vi "Defect Buddy 2014-09-20.vi"() -> ()   [LabVIEW 2010]
uses:
  <vilib>/addons/database/Connection.llb/Conn ObjectReference.ctl
  <vilib>/addons/database/_DB Variant To Data/Database Variant To Data.xnode
  <vilib>/addons/database/Connection.llb/DB Tools Open Connec (Path).vi
  <vilib>/addons/database/Connection.llb/Conn Execute.vi
  <vilib>/addons/database/Recordset.llb/Rec Fetch Recordset Data (R).vi
  <vilib>/addons/database/Recordset.llb/Rec Destroy - Connection.vi
  <vilib>/Utility/file.llb/Write To Spreadsheet File (string).vi
  <vilib>/addons/database/NI_Database_API.lvlib
  <vilib>/picture/3D Picture Control/NI_3D Picture Control.lvlib
panel:
  in  "Volumes":dbl[](array[numeric])=[5230.5515143, 4360.60278, 2309.371815, 7792.576126]
  in  "Markov-Payne Correction":bool
  out "Loaded Structure":T1={"Structure Name"="Batch6_3+111 Quasi-Bulk", "Lattice vector a"=[9.1641, 0.0, 0.0], "Lattice vector b"=[0.0, 7.93635, 0.0], "Lattice vector c"=[0.0, 0.0, 53.7091], "Atoms Array"=[{"Atom Name"="", "Positions (Direct)"=[[0.036896, 0.129554, 0.035254], [0.536896, 0.129554, 0.035254], [0.286896, 0.629554, 0.035254], [0.786896, 0.629554, 0.035254], [0.285415, 0.295133, 0.107673], [0.785415, 0.295133, 0.107673], [0.035415, 0.795133, 0.107673], [0.535415, 0.795133, 0.107673], [0.033615, 0.463308, 0.180101], [0.533615, 0.463308, 0.180101], [0.283615, 0.963308, 0.180101], [0.783615, 0.963308, 0.180101], [0.030844, 0.131453, 0.252535], [0.530844, 0.131453, 0.252535], [0.280844, 0.631453, 0.252535], [0.780844, 0.631453, 0.252535], [0.278379, 0.302058, 0.324923], [0.778379, 0.302058, 0.324923], [0.028379, 0.802058, 0.324923], [0.528379, 0.802058, 0.324923], [0.031198, 0.471844, 0.397363], [0.531198, 0.471844, 0.397363], [0.281198, 0.971844, 0.397363], [0.781198, 0.971844, 0.397363], [0.03247, 0.140643, 0.469814], [0.53247, 0.140643, 0.469814], [0.28247, 0.640643, 0.469814], [0.78247, 0.640643, 0.469814], [0.284308, 0.303948, 0.542263], [0.784308, 0.303948, 0.542263], [0.034308, 0.803948, 0.542263], [0.534308, 0.803948, 0.542263], [0.035944, 0.468219, 0.614701], [0.535944, 0.468219, 0.614701], [0.285944, 0.968219, 0.614701], [0.785944, 0.968219, 0.614701], [0.037813, 0.131858, 0.687216], [0.537813, 0.131858, 0.687216], [0.787813, 0.631858, 0.687216], [0.287813, 0.631858, 0.687216], [0.038238, 0.463759, 0.759817], [0.538238, 0.463759, 0.759817], [0.288238, 0.963758, 0.759817], [0.788238, 0.963758, 0.759817], [0.038639, 0.130134, 0.831025], [0.538639, 0.130134, 0.831025], [0.288639, 0.630134, 0.831025], [0.788639, 0.630134, 0.831025], [0.285712, 0.295024, 0.89873], [0.785712, 0.295024, 0.89873], [0.035712, 0.795024, 0.89873], [0.535712, 0.795024, 0.89873], [0.032596, 0.464879, 0.966384], [0.532596, 0.464879, 0.966384], [0.282596, 0.964879, 0.966384], [0.782596, 0.964879, 0.966384]], "Positions (Cartesian)"=[[0.33811863359999994, 1.0281858879, 1.8934606114], [4.9201686336, 1.0281858879, 1.8934606114], [2.6291436335999996, 4.9963608879, 1.8934606114], [7.2111936336, 4.9963608879, 1.8934606114], [2.6155716014999997, 2.34227878455, 5.7830199243000004], [7.197621601499999, 2.34227878455, 5.7830199243000004], [0.3245466015, 6.31045378455, 5.7830199243000004], [4.9065966014999995, 6.31045378455, 5.7830199243000004], [0.30805122149999997, 3.6769744458, 9.673062619100001], [4.890101221499999, 3.6769744458, 9.673062619100001], [2.5990762215, 7.6451494458, 9.673062619100001], [7.1811262215, 7.6451494458, 9.673062619100001], [0.2826575004, 1.04325701655, 13.5634275685], [4.8647075004, 1.04325701655, 13.5634275685], [2.5736825004, 5.011432016550001, 13.5634275685], [7.155732500399999, 5.011432016550001, 13.5634275685], [2.5510929938999998, 2.3972380083, 17.4513218993], [7.1331429939, 2.3972380083, 17.4513218993], [0.2600679939, 6.3654130083, 17.4513218993], [4.8421179939000005, 6.3654130083, 17.4513218993], [0.28590159179999997, 3.7447191294, 21.3420091033], [4.867951591799999, 3.7447191294, 21.3420091033], [2.5769265918, 7.7128941294, 21.3420091033], [7.158976591799999, 7.7128941294, 21.3420091033], [0.29755832699999996, 1.11619207305, 25.2332871074], [4.879608327, 1.11619207305, 25.2332871074], [2.588583327, 5.08436707305, 25.2332871074], [7.170633327, 5.08436707305, 25.2332871074], [2.6054269428, 2.4122377098, 29.124457693300002], [7.1874769428, 2.4122377098, 29.124457693300002], [0.31440194279999994, 6.3804127098, 29.124457693300002], [4.8964519428, 6.3804127098, 29.124457693300002], [0.32939441039999995, 3.71594986065, 33.0150374791], [4.9114444104, 3.71594986065, 33.0150374791], [2.6204194104, 7.684124860650001, 33.0150374791], [7.202469410399999, 7.684124860650001, 33.0150374791], [0.3465221133, 1.0464712383, 36.909752865600005], [4.9285721133, 1.0464712383, 36.909752865600005], [7.2195971133, 5.0146462383, 36.909752865600005], [2.6375471132999997, 5.0146462383, 36.909752865600005], [0.3504168558, 3.6805537396499997, 40.809087234699994], [4.9324668557999995, 3.6805537396499997, 40.809087234699994], [2.6414418557999997, 7.6487208033, 40.809087234699994], [7.2234918558, 7.6487208033, 40.809087234699994], [0.35409165989999997, 1.0327889709, 44.6336048275], [4.9361416599, 1.0327889709, 44.6336048275], [2.6451166599, 5.0009639709, 44.6336048275], [7.227166659899999, 5.0009639709, 44.6336048275], [2.6182933392, 2.3414137224, 48.269979443000004], [7.200343339199999, 2.3414137224, 48.269979443000004], [0.3272683392, 6.3095887224, 48.269979443000004], [4.9093183391999995, 6.3095887224, 48.269979443000004], [0.29871300359999997, 3.6894424516499997, 51.9036148944], [4.880763003599999, 3.6894424516499997, 51.9036148944], [2.5897380036, 7.65761745165, 51.9036148944], [7.171788003599999, 7.65761745165, 51.9036148944]]}, {"Atom Name"="", "Positions (Direct)"=[[0.286795, 0.296109, 0.054458], [0.786795, 0.296109, 0.054458], [0.036795, 0.796109, 0.054458], [0.536795, 0.796109, 0.054458], [0.035258, 0.462031, 0.126878], [0.535258, 0.462031, 0.126878], [0.285258, 0.962031, 0.126878], [0.785258, 0.962031, 0.126878], [0.033445, 0.130094, 0.199309], [0.533445, 0.130094, 0.199309], [0.283445, 0.630094, 0.199309], [0.783445, 0.630094, 0.199309], [0.280766, 0.298203, 0.27171], [0.780766, 0.298203, 0.27171], [0.030766, 0.798203, 0.27171], [0.530766, 0.798203, 0.27171], [0.028505, 0.468822, 0.344121], [0.528505, 0.468822, 0.344121], [0.278505, 0.968822, 0.344121], [0.778505, 0.968822, 0.344121], [0.03126, 0.138635, 0.416572], [0.53126, 0.138635, 0.416572], [0.28126, 0.638635, 0.416572], [0.78126, 0.638635, 0.416572], [0.282556, 0.307128, 0.489026], [0.782556, 0.307128, 0.489026], [0.032556, 0.807128, 0.489026], [0.532556, 0.807128, 0.489026], [0.034374, 0.470438, 0.56147], [0.534374, 0.470438, 0.56147], [0.284374, 0.970438, 0.56147], [0.784374, 0.970438, 0.56147], [0.035964, 0.134698, 0.633895], [0.535964, 0.134698, 0.633895], [0.285964, 0.634698, 0.633895], [0.785964, 0.634698, 0.633895], [0.037794, 0.465111, 0.706493], [0.537794, 0.465111, 0.706493], [0.787794, 0.965111, 0.706493], [0.287794, 0.965111, 0.706493], [0.038181, 0.130274, 0.779081], [0.538181, 0.130274, 0.779081], [0.288181, 0.630273, 0.779081], [0.788181, 0.630273, 0.779081], [0.288548, 0.296604, 0.847022], [0.788548, 0.296604, 0.847022], [0.038548, 0.796604, 0.847022], [0.538548, 0.796604, 0.847022], [0.035661, 0.461866, 0.914714], [0.535661, 0.461866, 0.914714], [0.285661, 0.961866, 0.914714], [0.785661, 0.961866, 0.914714], [0.032517, 0.131341, 0.982331], [0.532517, 0.131341, 0.982331], [0.282517, 0.631341, 0.982331], [0.782517, 0.631341, 0.982331]], "Positions (Cartesian)"=[[2.6282180595, 2.35002466215, 2.9248901678], [7.2102680595, 2.35002466215, 2.9248901678], [0.3371930595, 6.31819966215, 2.9248901678], [4.9192430595, 6.31819966215, 2.9248901678], [0.32310783779999996, 3.66683972685, 6.814503189799999], [4.9051578378, 3.66683972685, 6.814503189799999], [2.6141328378, 7.63501472685, 6.814503189799999], [7.1961828377999995, 7.63501472685, 6.814503189799999], [0.3064933245, 1.0324715168999998, 10.704707011899998], [4.8885433245, 1.0324715168999998, 10.704707011899998], [2.5975183244999998, 5.000646516900001, 10.704707011899998], [7.179568324499999, 5.000646516900001, 10.704707011899998], [2.5729677006, 2.36664337905, 14.593299561], [7.155017700599999, 2.36664337905, 14.593299561], [0.2819427006, 6.33481837905, 14.593299561], [4.863992700599999, 6.33481837905, 14.593299561], [0.2612226705, 3.7207354797, 18.4824292011], [4.843272670499999, 3.7207354797, 18.4824292011], [2.5522476705, 7.6889104797, 18.4824292011], [7.1342976705, 7.6889104797, 18.4824292011], [0.286469766, 1.1002558822500002, 22.3737072052], [4.8685197659999995, 1.1002558822500002, 22.3737072052], [2.577494766, 5.0684308822499995, 22.3737072052], [7.159544765999999, 5.0684308822499995, 22.3737072052], [2.5893714396, 2.4374753028000002, 26.2651463366], [7.1714214396, 2.4374753028000002, 26.2651463366], [0.2983464396, 6.4056503028, 26.2651463366], [4.8803964396, 6.4056503028, 26.2651463366], [0.3150067734, 3.7335606213, 30.156048377], [4.8970567734, 3.7335606213, 30.156048377], [2.6060317734, 7.7017356213, 30.156048377], [7.1880817733999995, 7.7017356213, 30.156048377], [0.3295776924, 1.0690104723, 34.045929944499996], [4.9116276924, 1.0690104723, 34.045929944499996], [2.6206026924, 5.0371854723, 34.045929944499996], [7.202652692399999, 5.0371854723, 34.045929944499996], [0.3463479954, 3.69128368485, 37.9451031863], [4.928397995399999, 3.69128368485, 37.9451031863], [7.2194229953999995, 7.659458684850001, 37.9451031863], [2.6373729954, 7.659458684850001, 37.9451031863], [0.34989450209999995, 1.0339000599000001, 41.843739337100004], [4.9319445020999995, 1.0339000599000001, 41.843739337100004], [2.6409195021, 5.00206712355, 41.843739337100004], [7.2229695021, 5.00206712355, 41.843739337100004], [2.6442827268, 2.3539531553999997, 45.4927893002], [7.2263327268, 2.3539531553999997, 45.4927893002], [0.35325772679999995, 6.3221281554, 45.4927893002], [4.9353077268, 6.3221281554, 45.4927893002], [0.3268009701, 3.6655302291, 49.1284656974], [4.9088509701000005, 3.6655302291, 49.1284656974], [2.6178259700999997, 7.6337052291, 49.1284656974], [7.1998759701, 7.6337052291, 49.1284656974], [0.29798903969999996, 1.04236814535, 52.760113912099996], [4.8800390397, 1.04236814535, 52.760113912099996], [2.5890140397, 5.010543145350001, 52.760113912099996], [7.1710640397, 5.010543145350001, 52.760113912099996]]}], "# of atoms"=112}
  out "Indicies":cluster{i32, i32}[](array[cluster])
  out "All Hosts and Defects":T2(array[cluster])
  out "Transitions":T3(array[cluster])
  out "Thermodynamic Fermi Level (eV)":dbl
  out "Defects to Bind":i32[](array[numeric])
  in  "Plot Binding Energy":bool
  in  "Calc Thermodynamic Fermi Level":bool
  in  "Thermodynamic Fermi Level":i32
  in  "Color Array Type":T4(ring)=enum."Contrasting Colors"
  in  "Show Charge Transitions":bool=TRUE
  out "connection reference":T5
  in  "Plots Tab":T6(tab)
  in  "Make Awesome Looking":bool
  out "Te Rich Limit":cluster{dbl[], dbl[]}[](graph)
  out "Cd Rich Limit":cluster{"appended array":dbl[], dbl[]}[](graph)
  in  "Chemical Potential":dbl(slide) scale=0.0..1.0
  in  "Chemical Potential 2":dbl(slide)=1.0 scale=0.0..1.0
  in  "Save as a table":bool
  out "Te Rich Limit 2":cluster{dbl[], dbl[]}[](graph)
  out "Cd Rich Limit 2":cluster{"appended array":dbl[], dbl[]}[](graph)
  in  "Chemical Potential 5":dbl(slide) scale=0.0..1.0
  in  "Chemical Potential 3":dbl(slide)=1.0 scale=0.0..1.0
  in  "Save as a table 2":bool
  in  "Seperate Defects":i32(listbox)
  in  "Set as seperate defects":bool
  out "Binding Energy":cluster{"Array":dbl[], dbl[]}[](graph)
  in  "Binding Energy Chem Pot":dbl(slide) scale=0.0..1.0
  out "Defect Energy Levels":cluster{dbl[], dbl[]}[](graph)
  in  "Buckets":string[][](array[combo])
  in  "Load in VESTA":bool
  in  "Atomic Structures":i32(listbox)
  out "Atomic Structure":refnum<vi>(3d-picture)
  in  "Options":cluster{"Border?":bool, "Bonds?":bool}
  in  "Atom Size":dbl=0.75
  in  "Plot Atomic Structure":bool
  in  "Scale":dbl(slide)=0.07482993197278912 scale=0.0..0.5
  in  "Setup Camera":bool
  in  "Ignore Location":bool
  in  "Potential Re-alignment":bool
  out "Defects":T7(array[cluster])
  out "Base Object":refnum<vi>
  in  "VBM":dbl=1.79581
  in  "Pure Structures with defects":i32[](listbox)
  in  "Related Defects":i32[](listbox)
  in  "UDL":path=path "D:/Ab-initio/VASP Calcs/VASP DB.udl"
  # "Cd Rich"
  # "Te Rich"
  # "Cd Rich"
  # "Te Rich"
  # "p-type"
  # "n-type"
  # "p-type"
  # "n-type"
  # "Cd Rich"
  # "Te Rich"
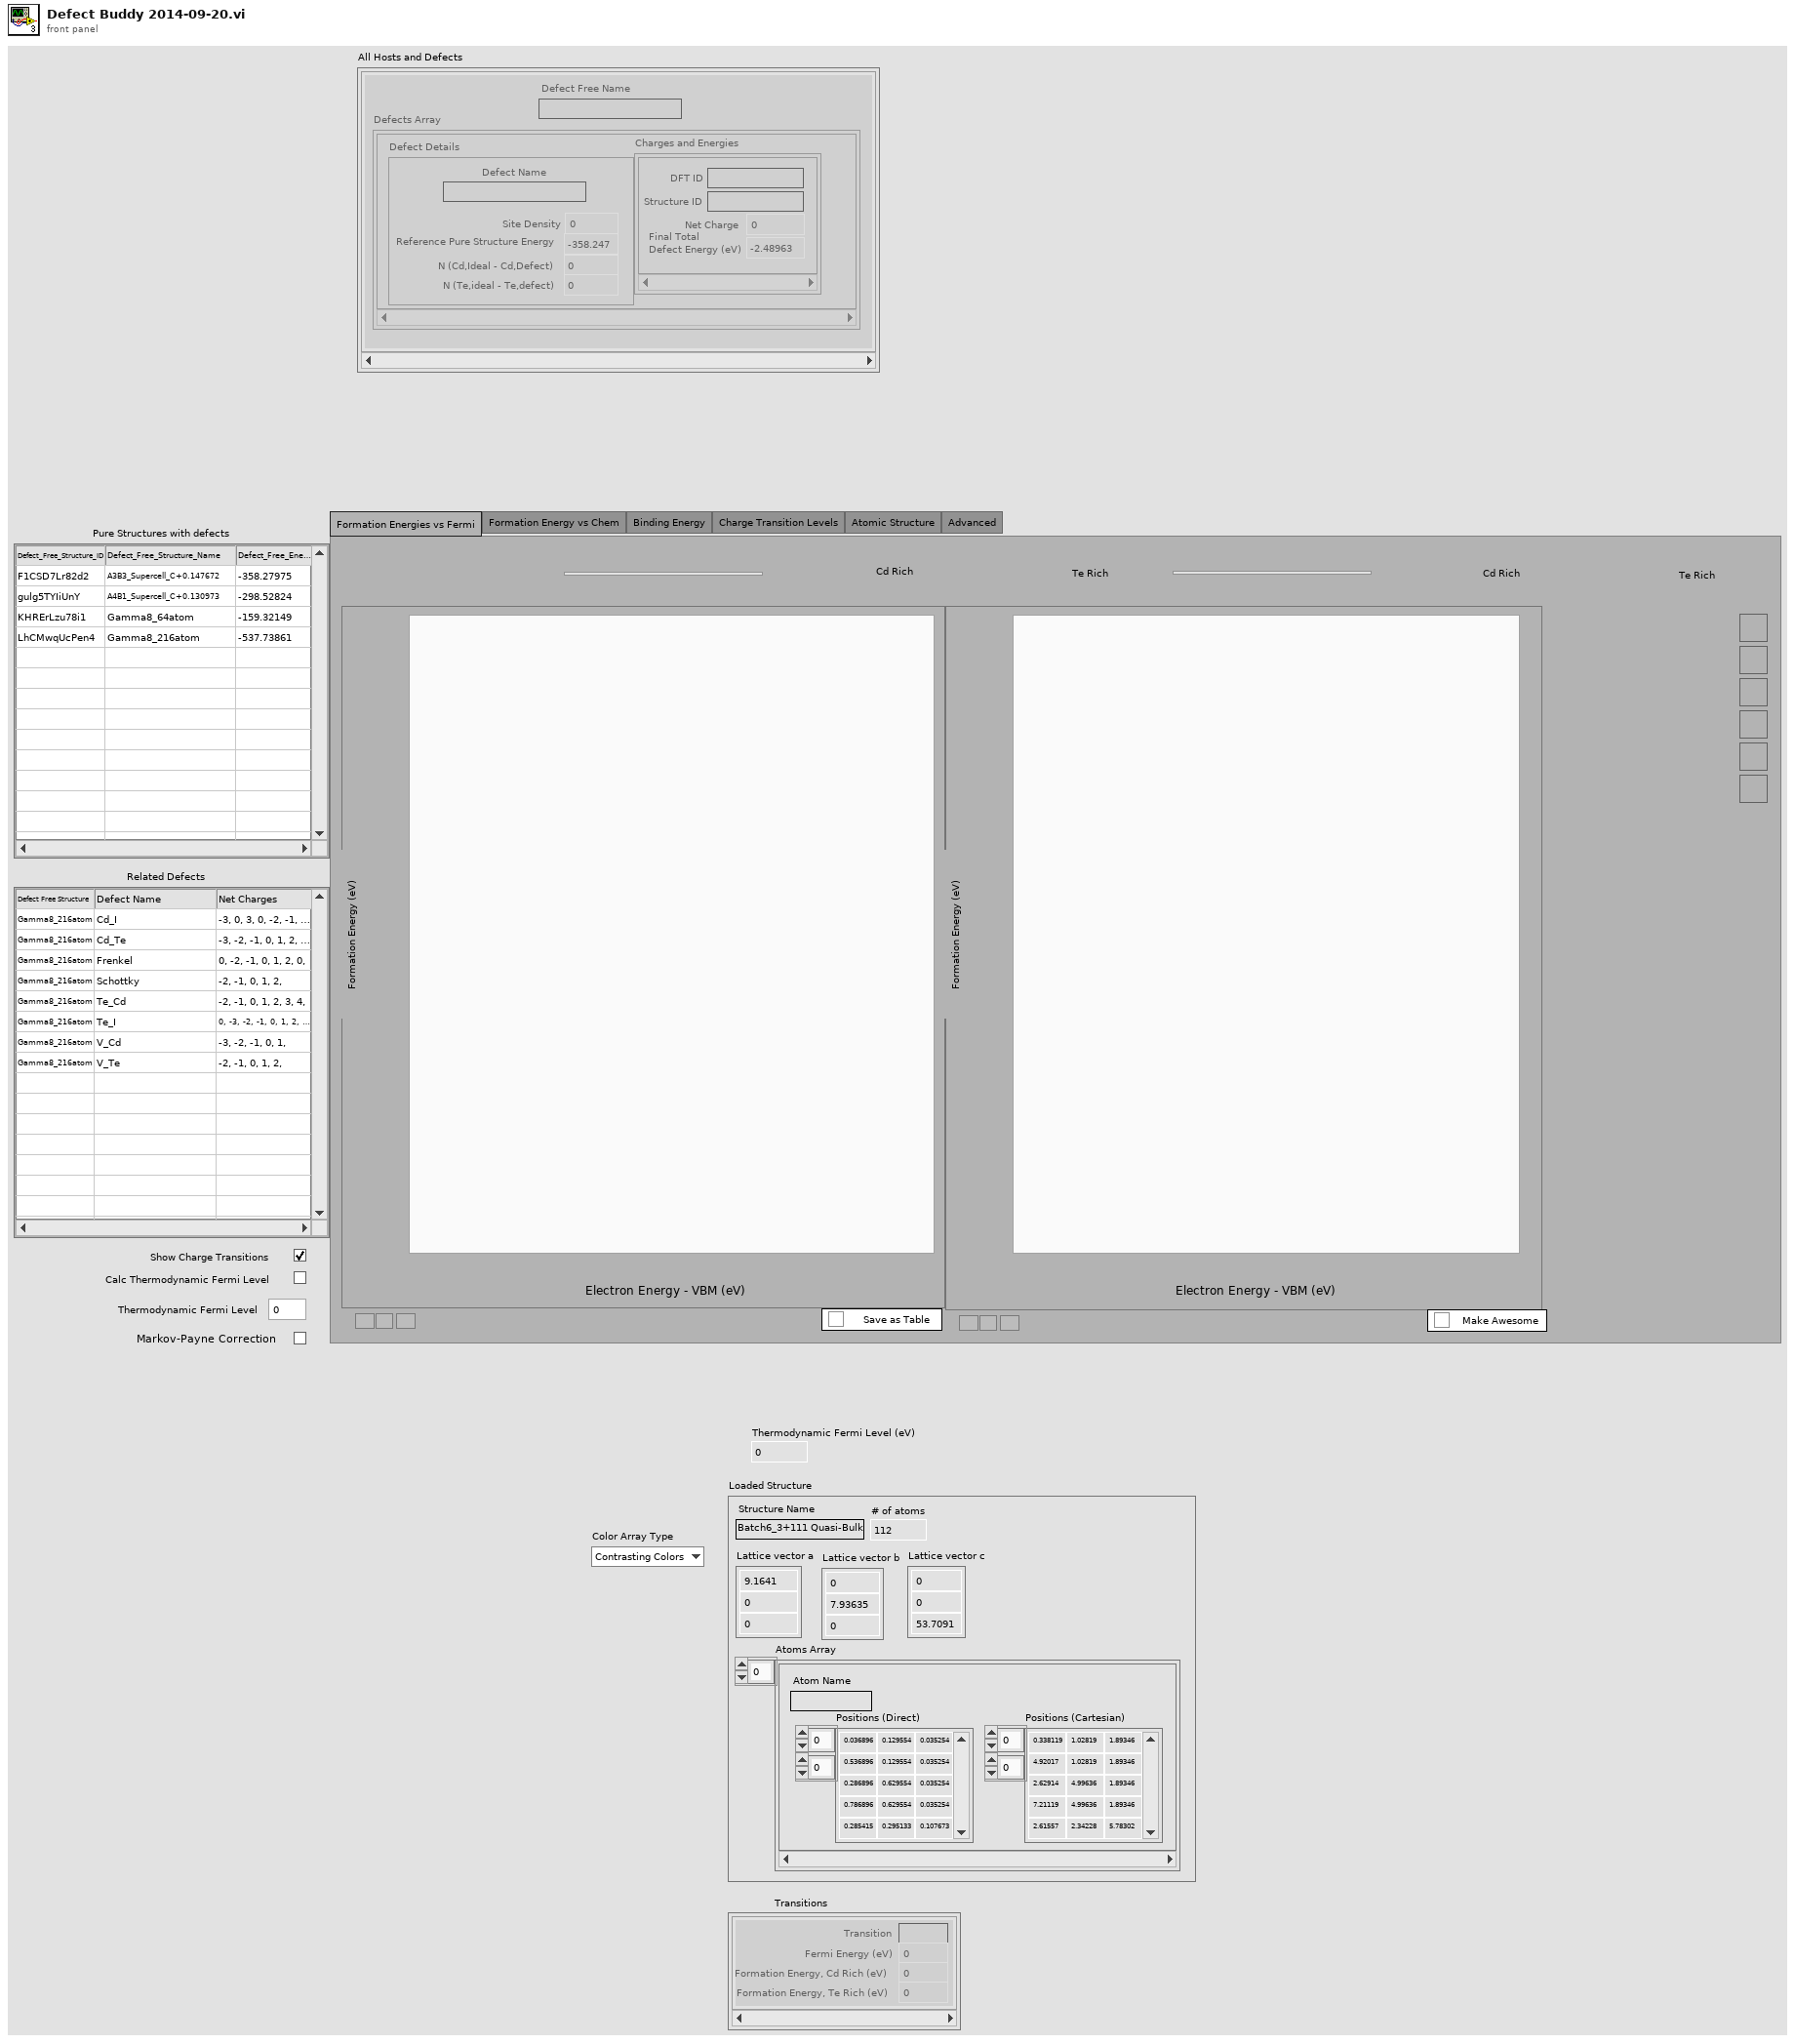
[diagram p1: front panel]
types:
  T1 = cluster{"Structure Name":string, "Lattice vector a":dbl[], "Lattice vector b":dbl[], "Lattice vector c":dbl[], "Atoms Array":cluster{"Atom Name":string, "Positions (Direct)":dbl[][], "Positions (Cartesian)":dbl[][]}[], "# of atoms":i32}
  T2 = cluster{"Defect Free Name":string, "Defects Array":cluster{"Defect Details":cluster{"Defect Name":string, "Site Density":dbl, "Reference Pure Structure Energy":dbl, "N (Cd,Ideal - Cd,Defect)":i32, "N (Te,ideal - Te,defect)":i32}, "Charges and Energies":cluster{"DFT ID":string, "Structure ID":string, "Net Charge":i32, "Final Total \nDefect Energy (eV)":dbl}[]}[]}[]
  T3 = cluster{"Transition":string, "Fermi Energy (eV)":dbl, "Formation Energy, Cd Rich (eV)":dbl, "Formation Energy, Te Rich (eV)":dbl}[]
  T4 = enum16{"Visible Spectrum", "Greyscale", "Contrasting Colors"}
  T5 = typedef "NI_Database_API.lvlib/Conn ObjectReference.ctl" = refnum<k1>
  T6 = enum32{"Formation Energies vs Fermi", "Formation Energy vs Chem", "Binding Energy", "Charge Transition Levels", "Atomic Structure", "Advanced"}
  T7 = cluster{"Defect Details":cluster{"Defect Name":string, "Site Density":dbl, "Reference Pure Structure Energy":dbl, "N (Cd,Ideal - Cd,Defect)":i32, "N (Te,ideal - Te,defect)":i32}, "Charges and Energies":cluster{"Net Charge":i32, "Final Total \nDefect Energy (eV)":dbl}[]}[]
  T8 = typedef "NI_Database_API.lvlib/Rec ObjectReference.ctl" = refnum<k1>
  T9 = cluster{"Name":string, "Color":u32, "Style":u8, "Point Style":u8, "Name Visible":bool, "Allow Drag":bool, "Annotation Mode":u32, "Plot":i32, "Index":i32, "Position":cluster{"X":dbl, "Y":dbl}, "X Scale":u32, "Y Scale":u32, "Show Arrow":bool, "Lock Name":bool, "Plot Area":i32, "Label Offset":cluster{"X":dbl, "Y":dbl}}
  T10 = cluster{"Name":string, "Color":u32, "Style":u8, "Point Style":u8, "Name Visible":bool, "Allow Drag":bool, "Cursor Mode":u32, "Plot":i32, "Index":i32, "Position":cluster{"X":dbl, "Y":dbl}, "X Scale":u32, "Y Scale":u32, "Watch Plots":i32[], "Watch All Plots":bool, "Plot Area":i32, "Label Offset":cluster{"X":dbl, "Y":dbl}}
  T11 = cluster{"Defect Details":cluster{"Defect Name":string, "Site Density":dbl, "Reference Pure Structure Energy":dbl, "N (Cd,Ideal - Cd,Defect)":i32, "N (Te,ideal - Te,defect)":i32}, "Charges and Energies":cluster{"DFT ID":string, "Structure ID":string, "Net Charge":i32, "Final Total \nDefect Energy (eV)":dbl}[]}[]
  T12 = cluster{"Defect Name":string, "Site Density":dbl, "Reference Pure Structure Energy":dbl, "N (Cd,Ideal - Cd,Defect)":i32, "N (Te,ideal - Te,defect)":i32}
  T13 = cluster{"DFT ID":string, "Structure ID":string, "Net Charge":i32, "Final Total \nDefect Energy (eV)":dbl}[]
  T14 = cluster{string, "Defects Array":cluster{"Defect Details":cluster{"Defect Name":string, "Site Density":dbl, "Reference Pure Structure Energy":dbl, "N (Cd,Ideal - Cd,Defect)":i32, "N (Te,ideal - Te,defect)":i32}, "Charges and Energies":cluster{"DFT ID":string, "Structure ID":string, "Net Charge":i32, "Final Total \nDefect Energy (eV)":dbl}[]}[]}
  T15 = cluster{"Name":string, "Color":u32, "Style":u8, "Point Style":u8, "Name Visible":bool, "Allow Drag":bool, "Cursor Mode":u32, "Plot":i32, "Index":i32, "Position":cluster{"X":dbl, "Y":dbl}, "X Scale":u32, "Y Scale":u32, "Watch Plots":i32[], "Watch All Plots":bool, "Plot Area":i32, "Label Offset":cluster{"X":dbl, "Y":dbl}}[]
  T16 = cluster{"Name":string, "Color":u32, "Style":u8, "Point Style":u8, "Name Visible":bool, "Allow Drag":bool, "Annotation Mode":u32, "Plot":i32, "Index":i32, "Position":cluster{"X":dbl, "Y":dbl}, "X Scale":u32, "Y Scale":u32, "Show Arrow":bool, "Lock Name":bool, "Plot Area":i32, "Label Offset":cluster{"X":dbl, "Y":dbl}}[]
  T17 = cluster{"Defect Free Name":string, "Defects Array":cluster{"Defect Details":cluster{"Defect Name":string, "Site Density":dbl, "Reference Pure Structure Energy":dbl, "N (Cd,Ideal - Cd,Defect)":i32, "N (Te,ideal - Te,defect)":i32}, "Charges and Energies":cluster{"DFT ID":string, "Structure ID":string, "Net Charge":i32, "Final Total \nDefect Energy (eV)":dbl}[]}[]}
  T18 = cluster{"Defect Details":cluster{"Defect Name":string, "Site Density":dbl, "Reference Pure Structure Energy":dbl, "N (Cd,Ideal - Cd,Defect)":i32, "N (Te,ideal - Te,defect)":i32}, "Charges and Energies":cluster{"DFT ID":string, "Structure ID":string, "Net Charge":i32, "Final Total \nDefect Energy (eV)":dbl}[]}
  T19 = cluster{"Defect Name":string, "Transitions":cluster{"Transition":string, "Fermi Energy (eV)":dbl, "Formation Energy, Cd Rich (eV)":dbl, "Formation Energy, Te Rich (eV)":dbl}[]}
  T20 = cluster{"Defect Name":string, "Transitions":cluster{"Transition":string, "Fermi Energy (eV)":dbl, "Formation Energy, Cd Rich (eV)":dbl, "Formation Energy, Te Rich (eV)":dbl}[]}[]
  T21 = cluster{"Lattice vector b[0]":dbl, "Lattice vector b[1]":dbl, "Lattice vector b[2]":dbl}
  T22 = typedef "LVAnnotationListTypeDef.ctl" = cluster{"Name":string, "Color":u32, "Style":u8, "Point Style":u8, "Name Visible":bool, "Allow Drag":bool, "Annotation Mode":u32, "Plot":i32, "Index":i32, "Position":cluster{"X":dbl, "Y":dbl}, "X Scale":u32, "Y Scale":u32, "Show Arrow":bool, "Lock Name":bool, "Plot Area":i32, "Label Offset":cluster{"X":dbl, "Y":dbl}}[]
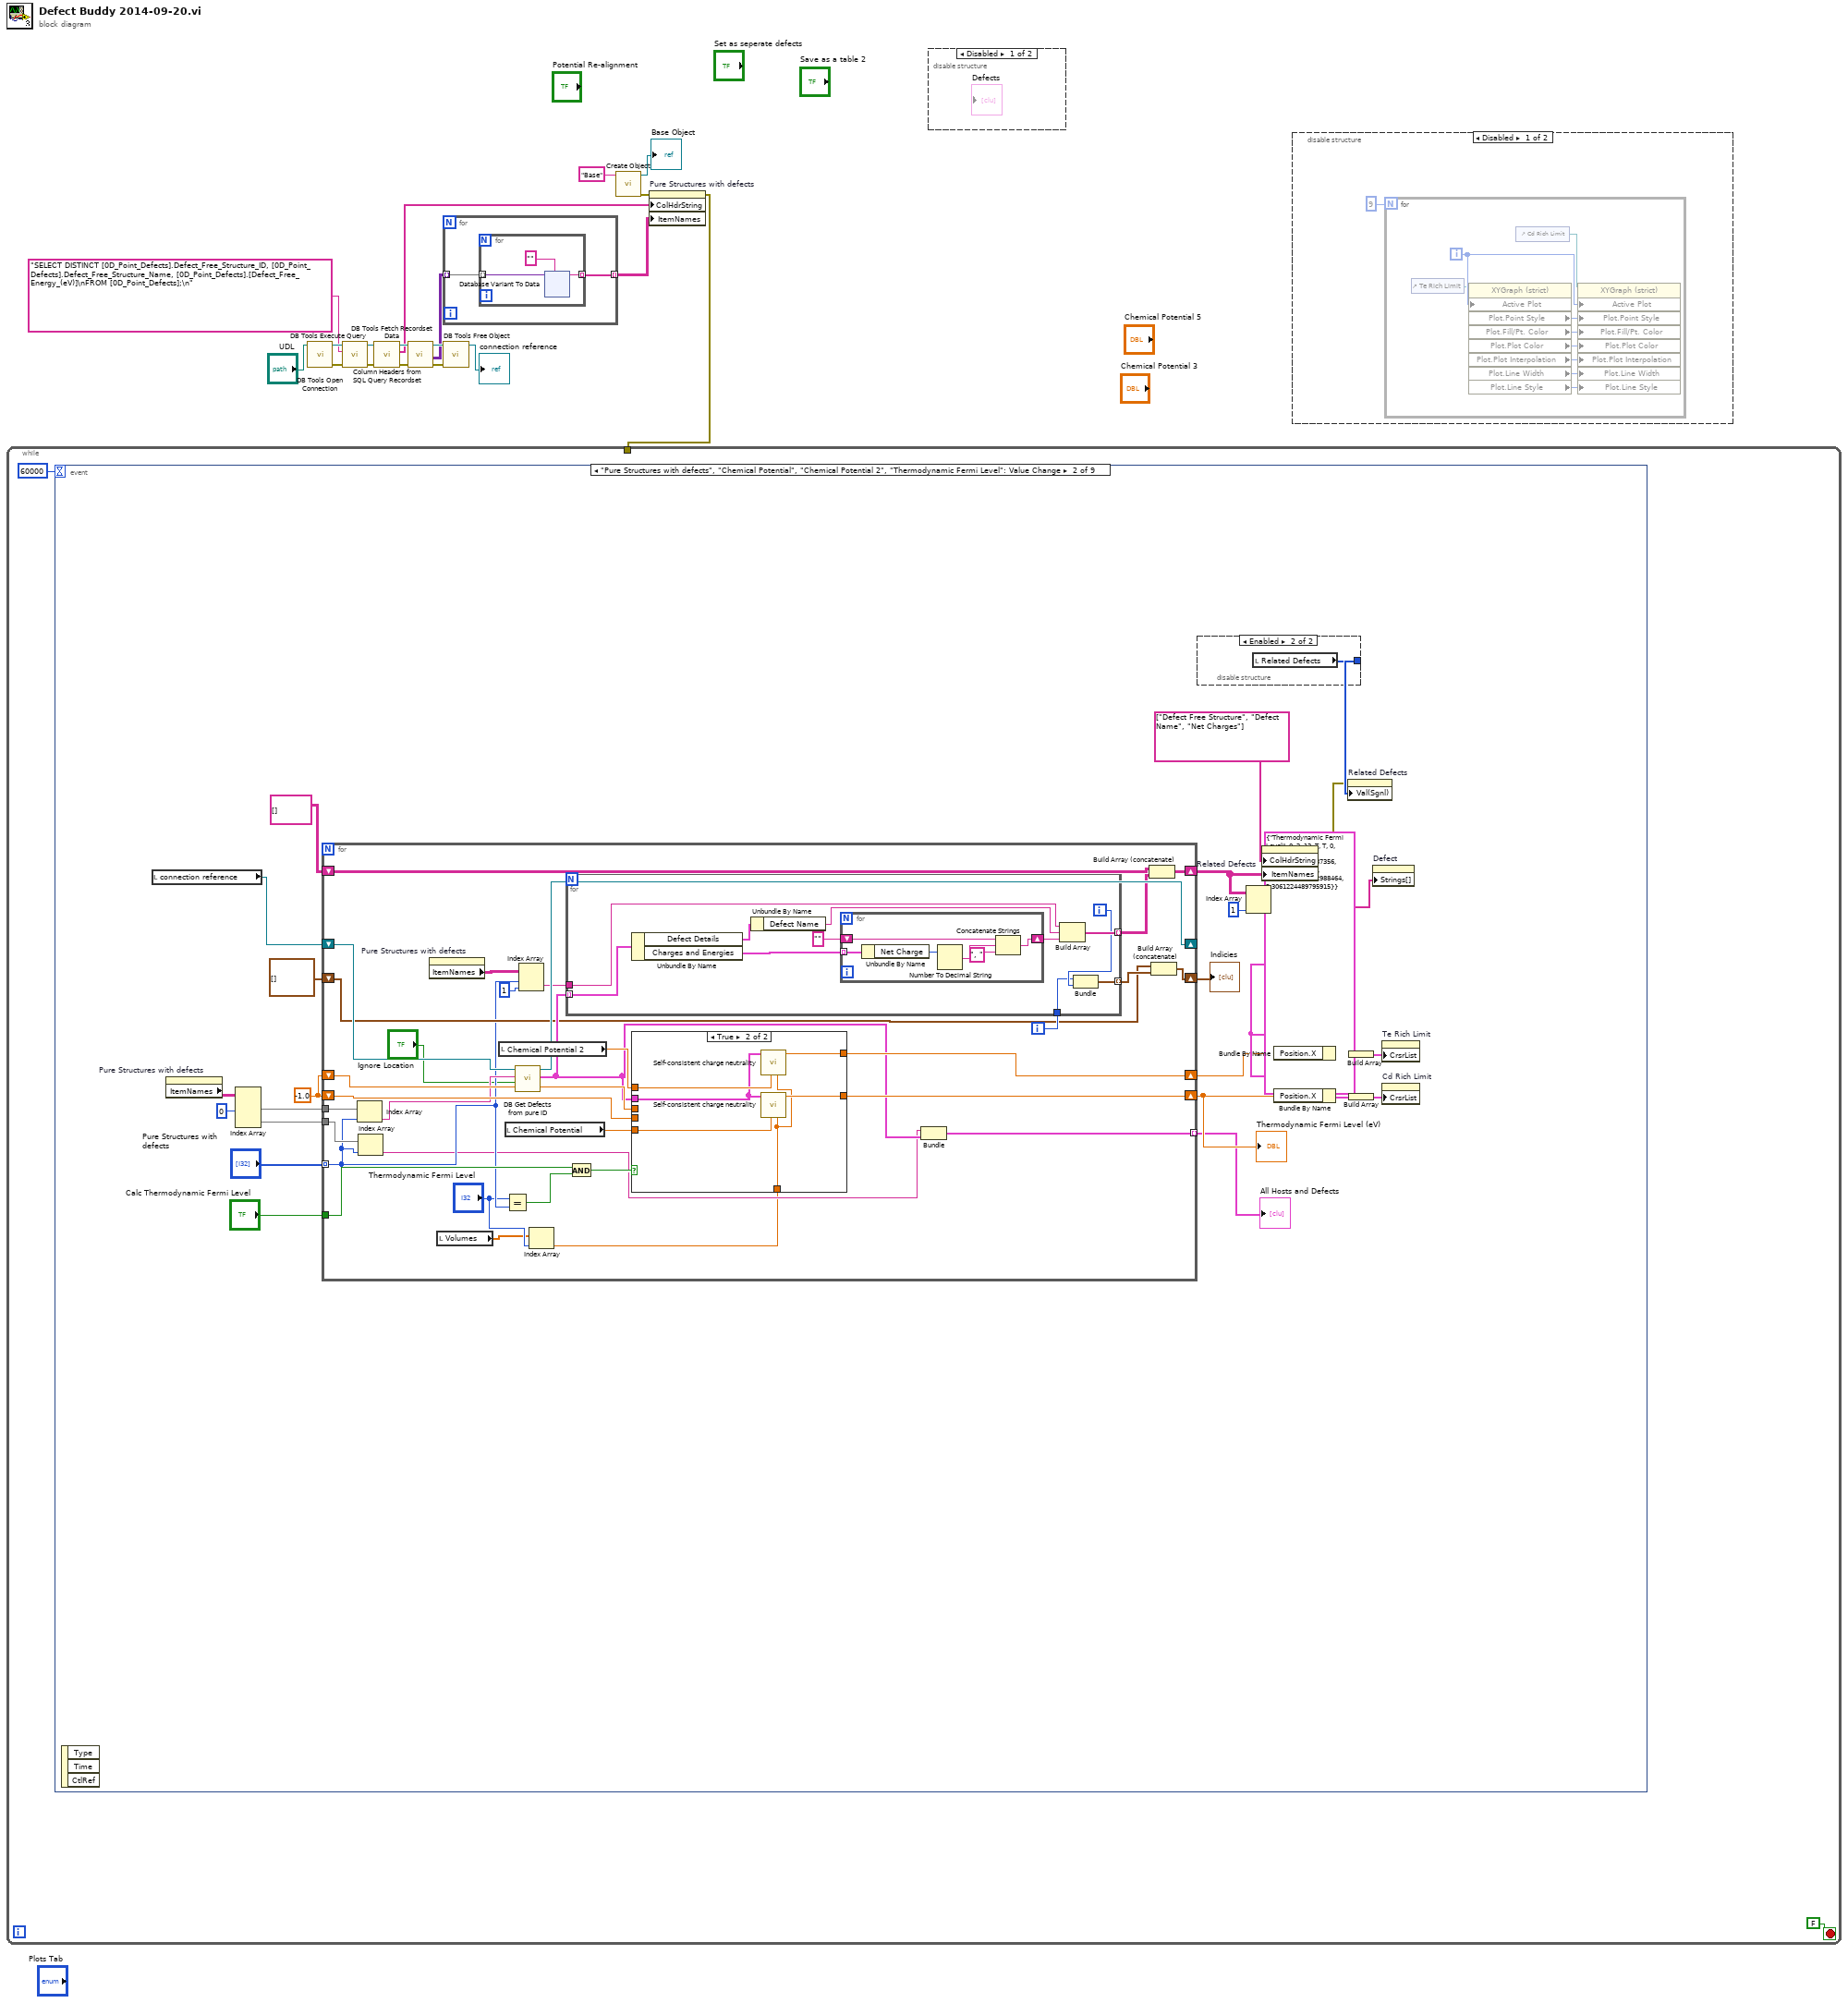
[diagram p0: block diagram]
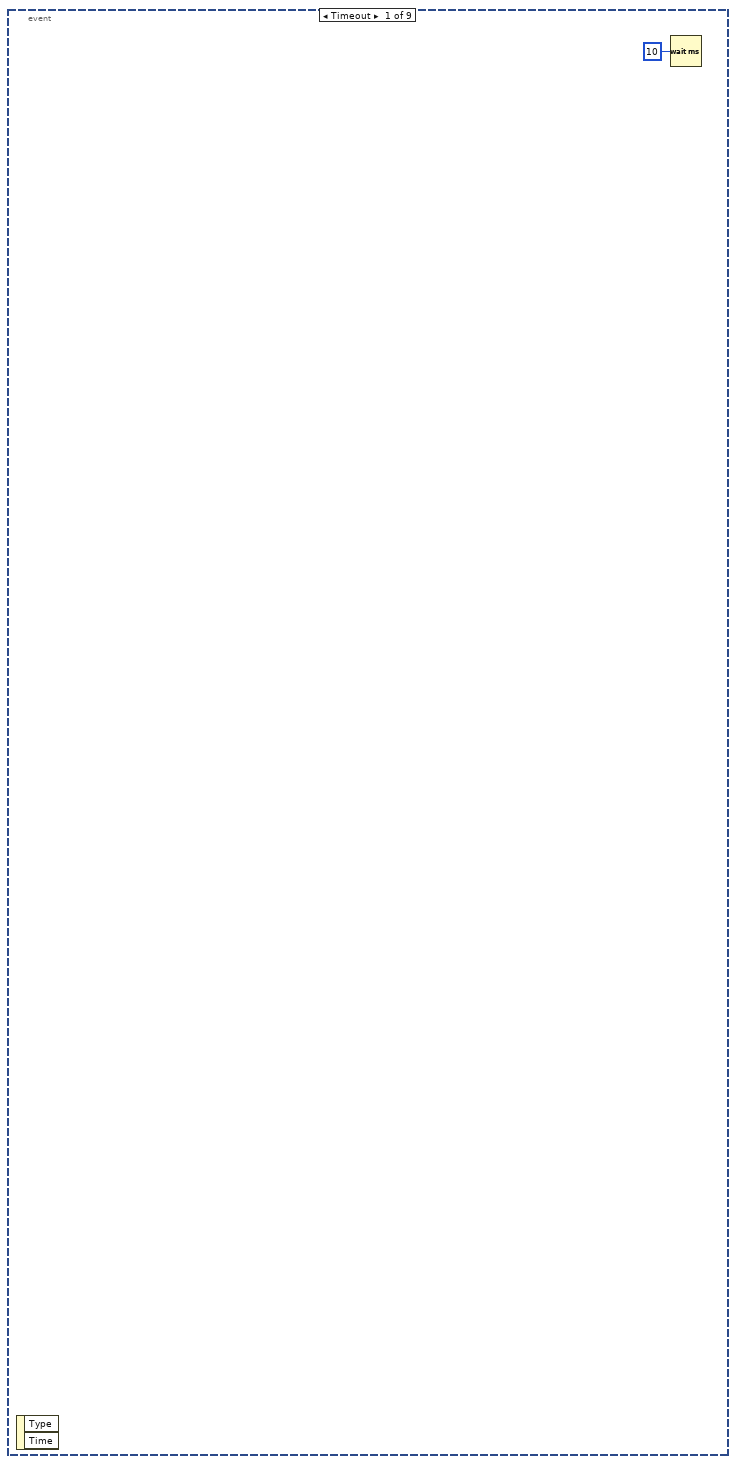
[diagram p4: hidden frame]
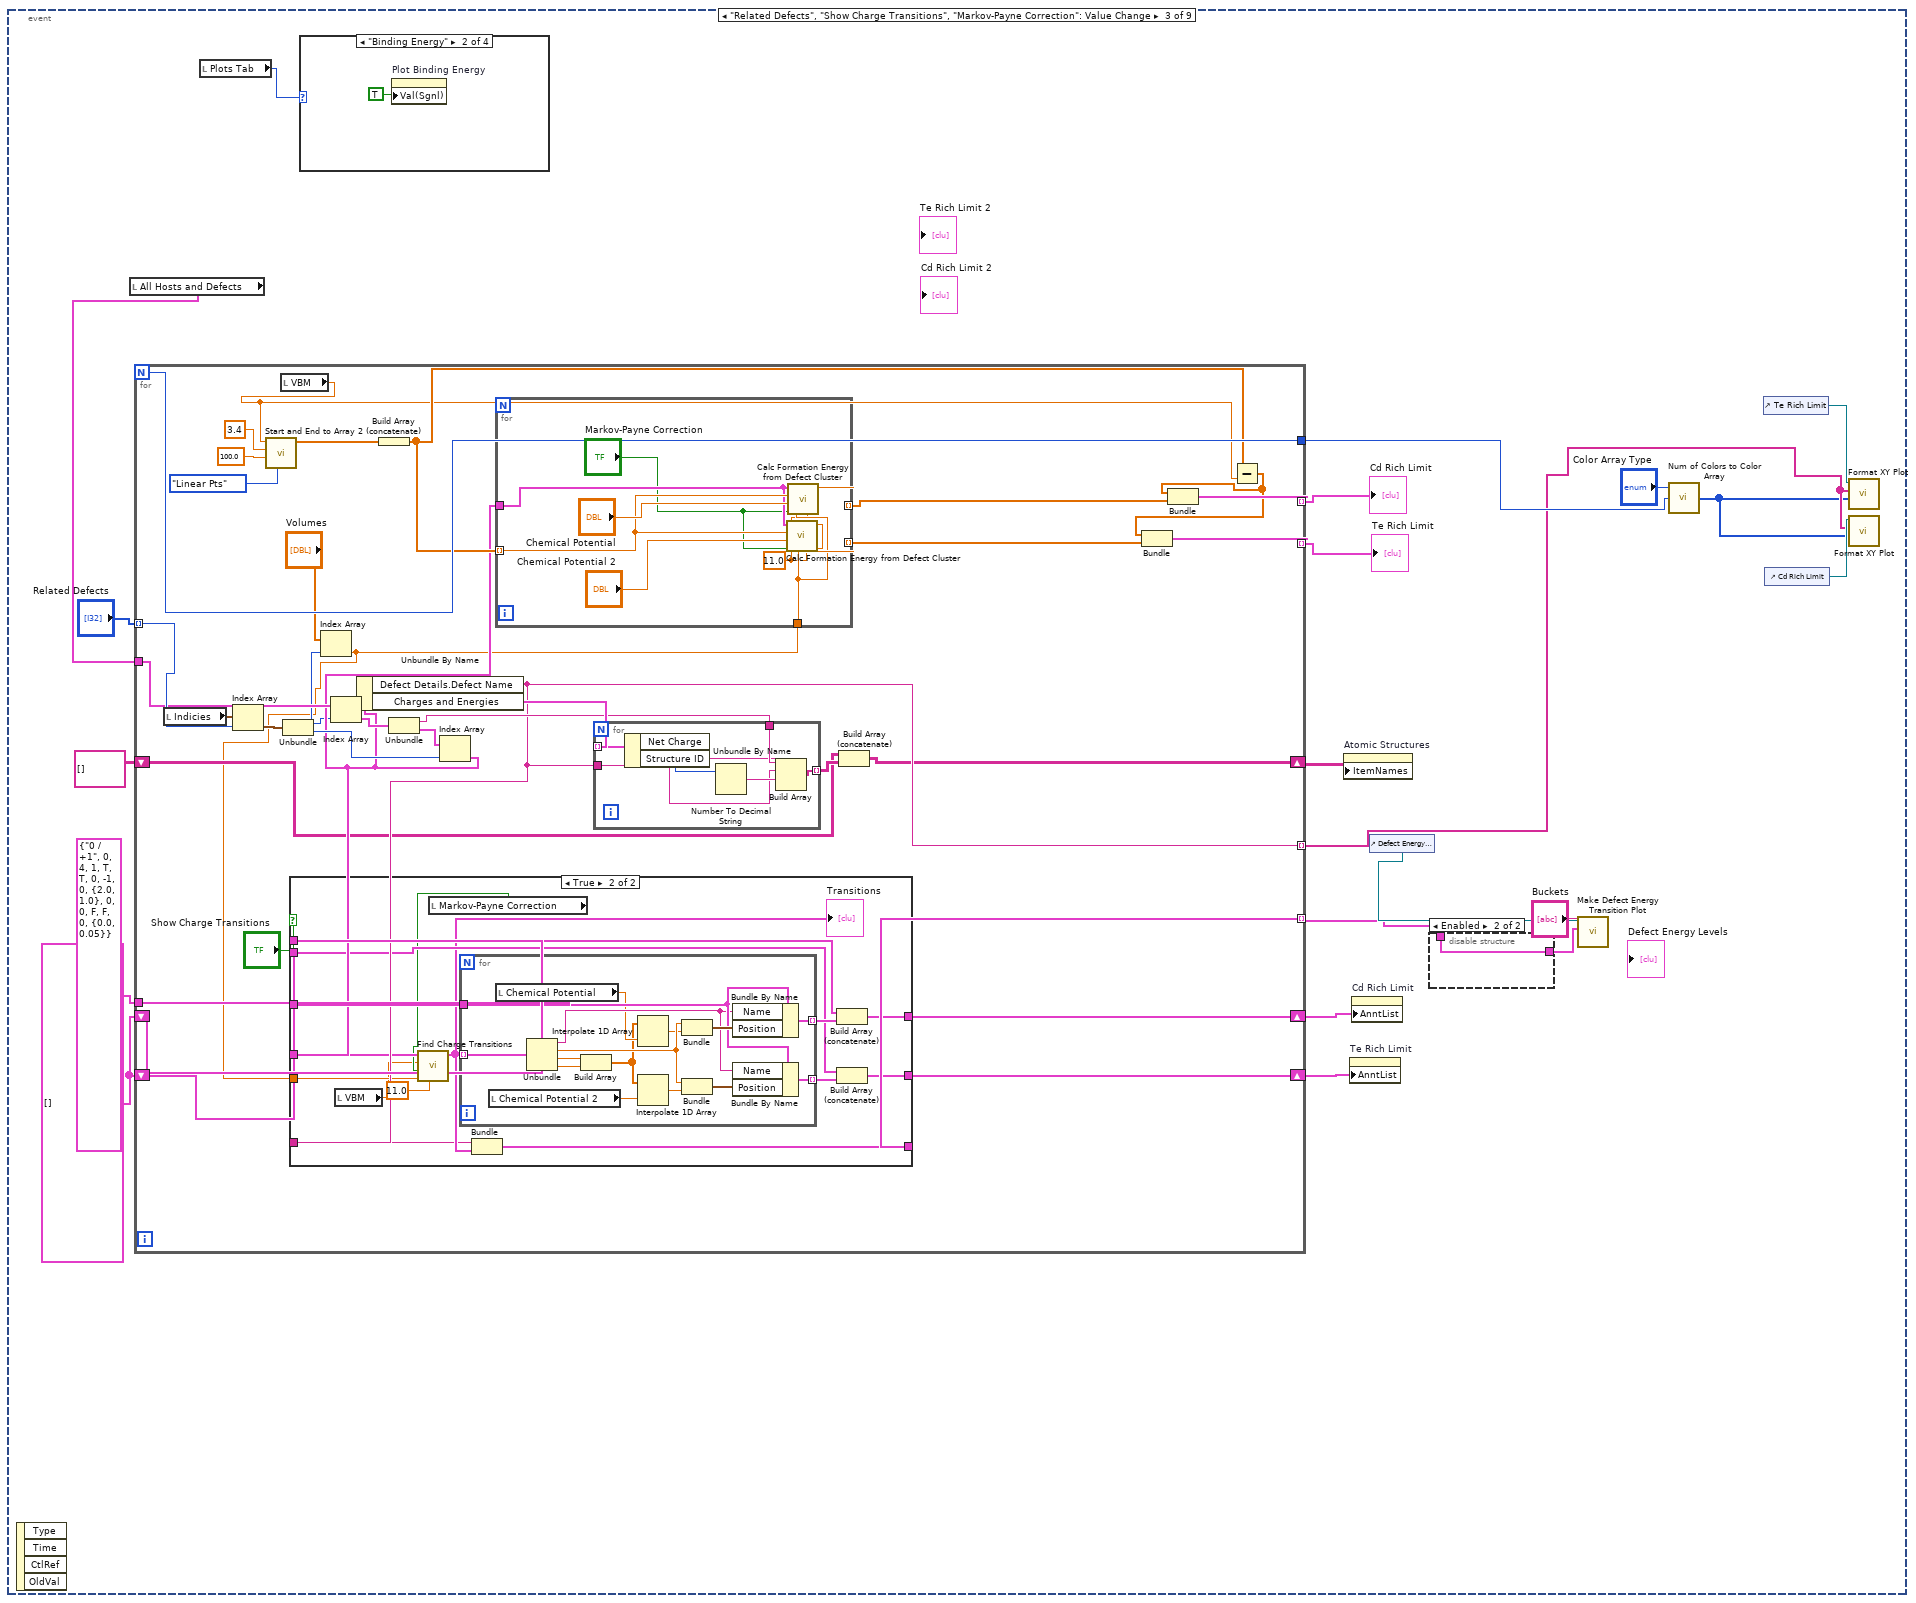
[diagram p7: hidden frame]
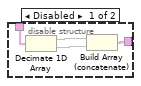
[diagram p8: hidden frame]
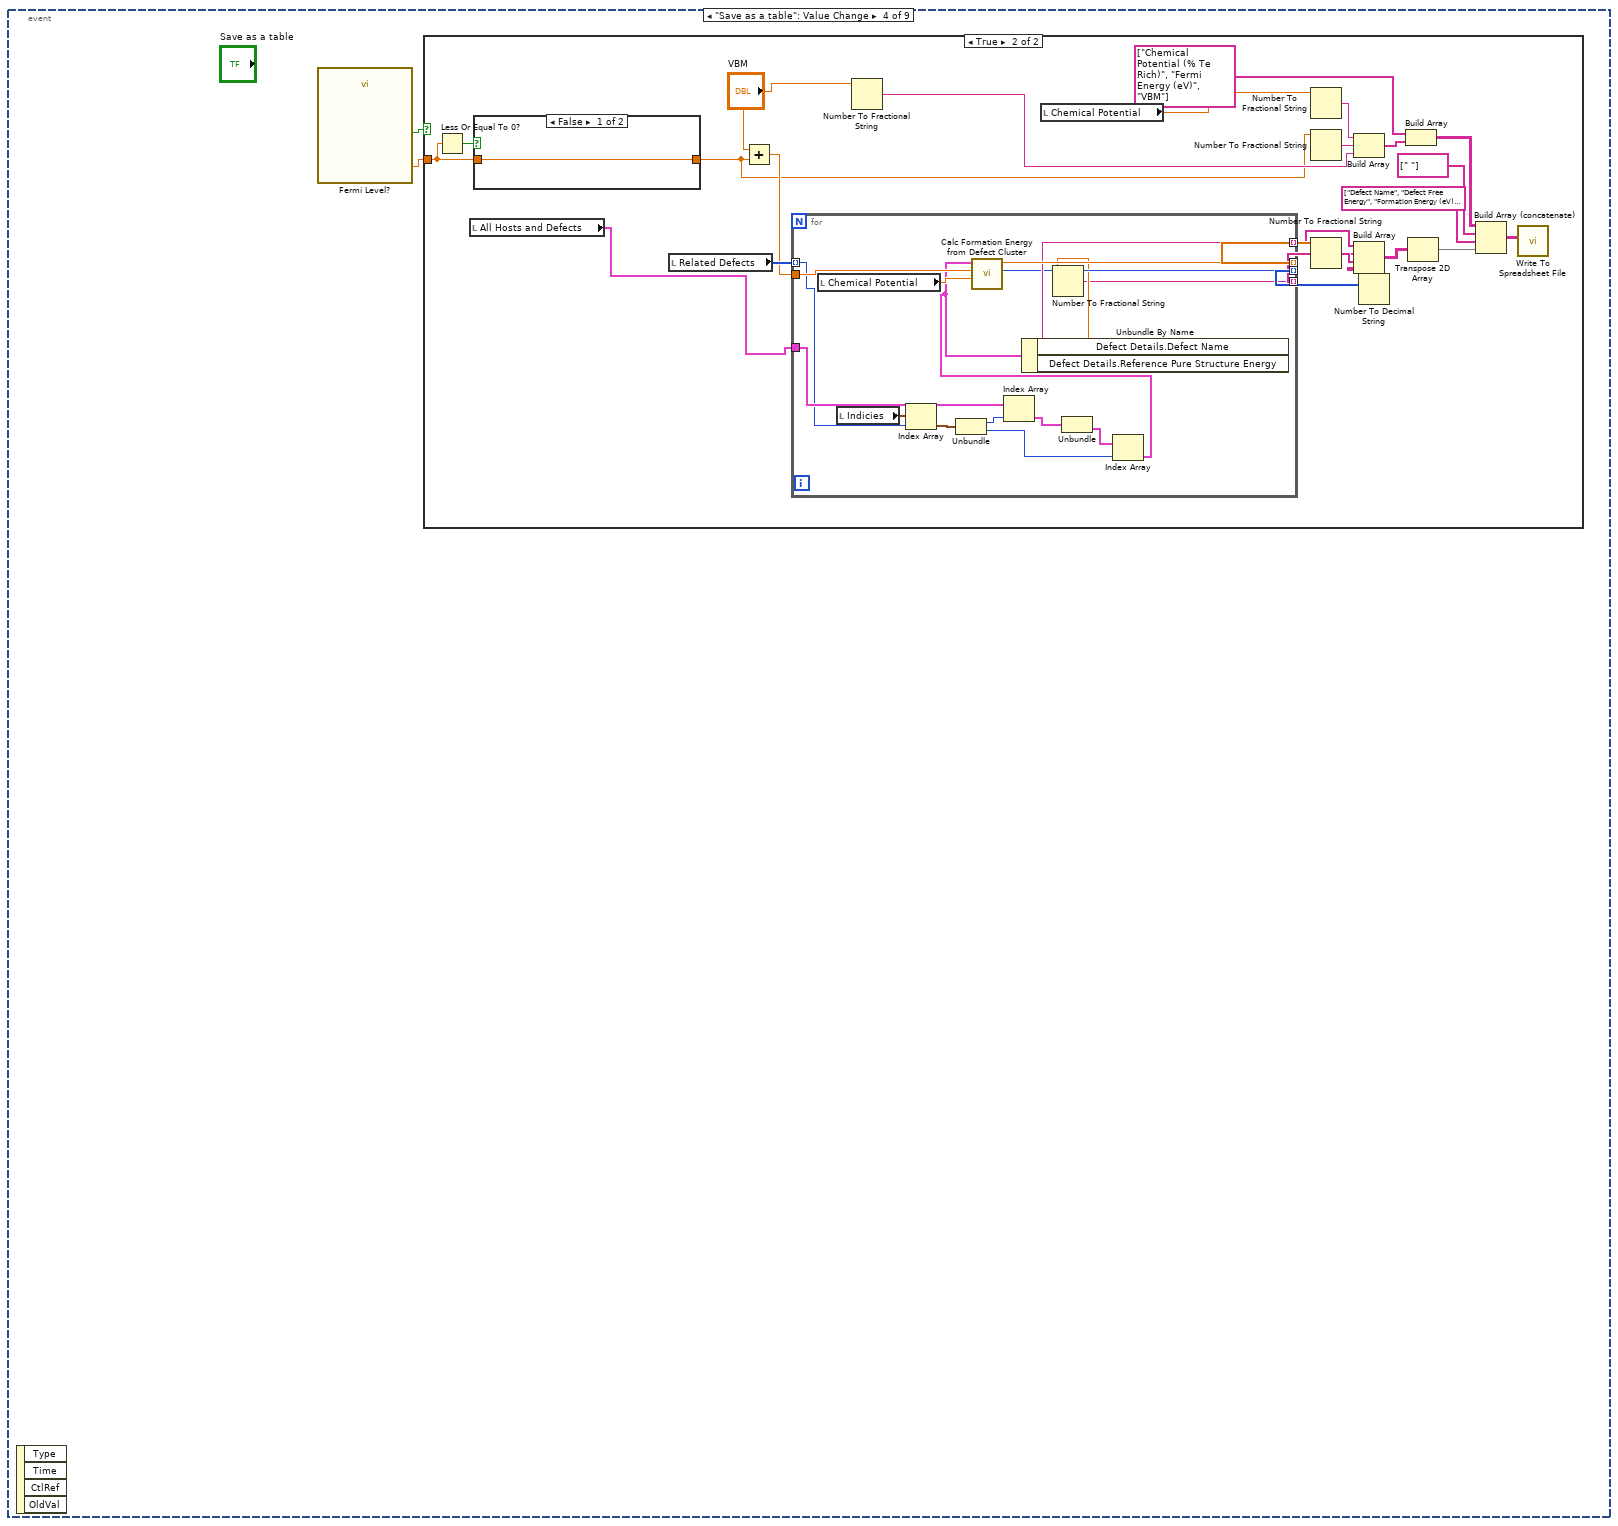
[diagram p13: hidden frame]
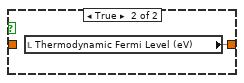
[diagram p15: hidden frame]
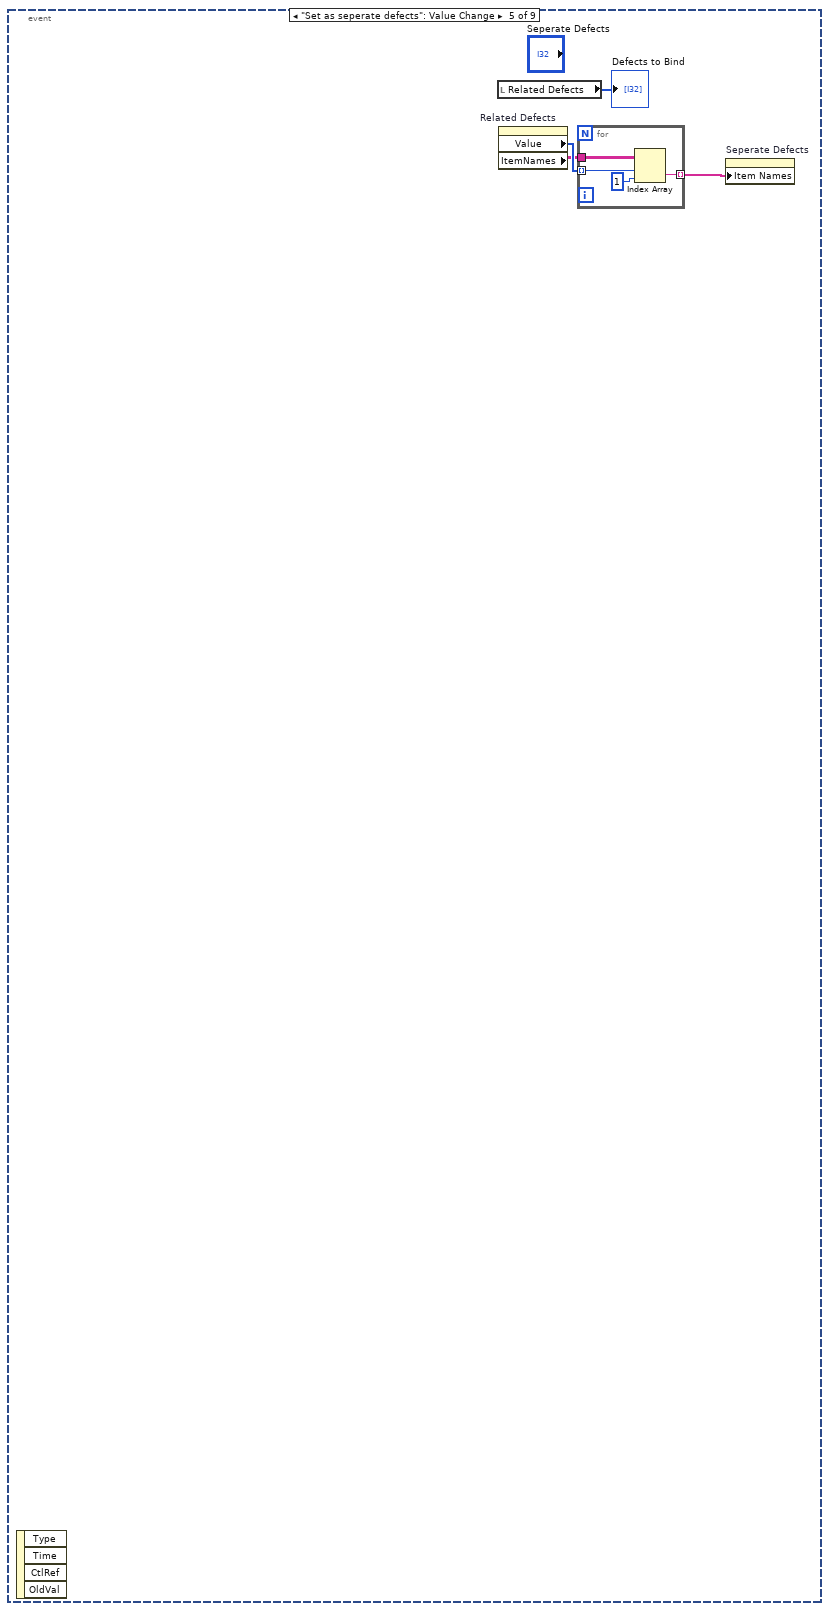
[diagram p16: hidden frame]
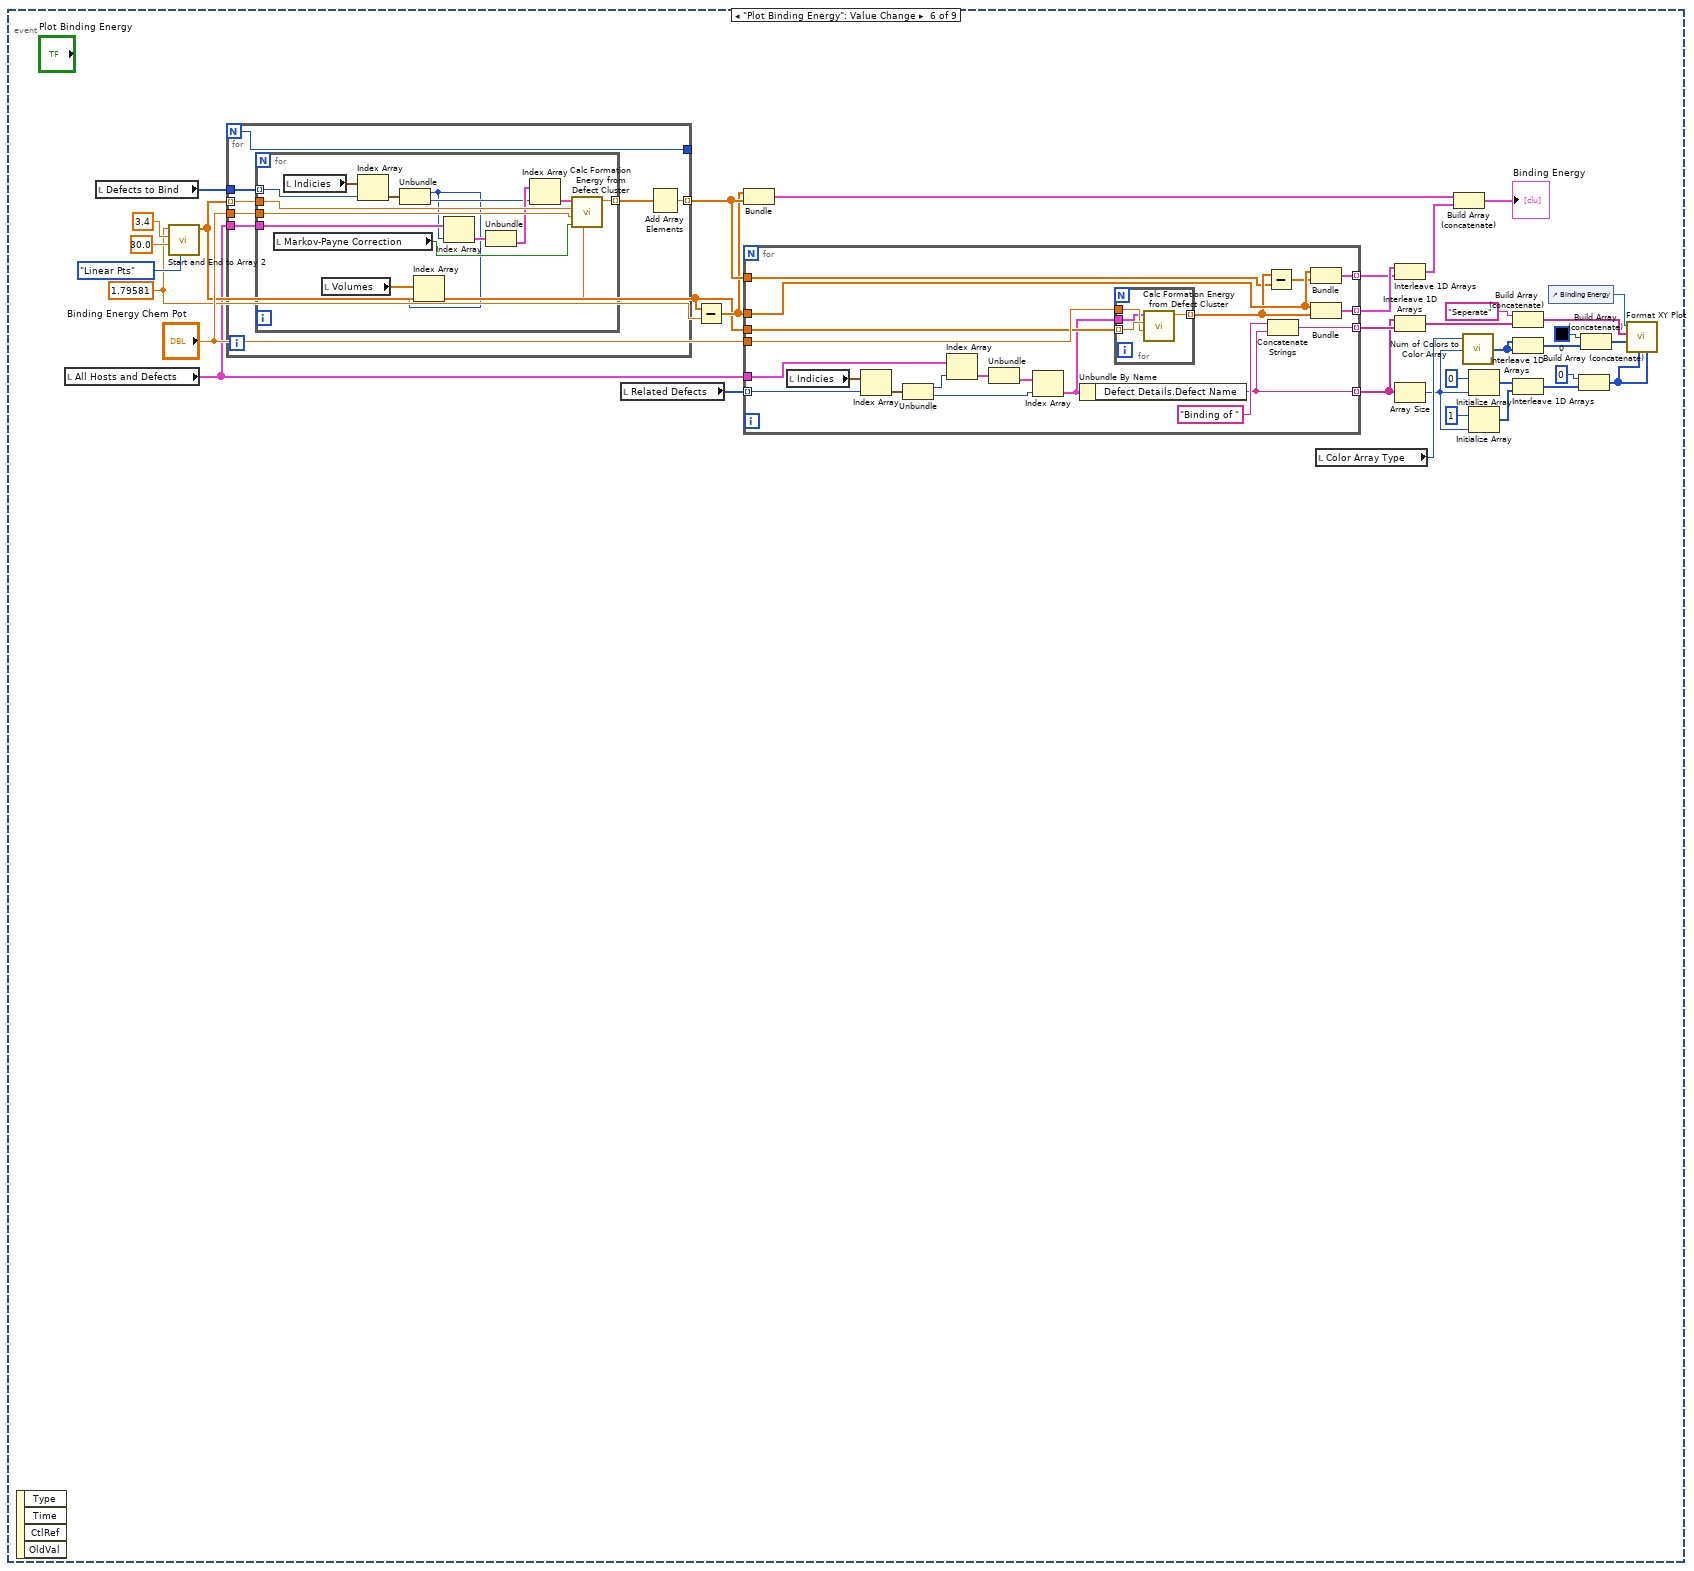
[diagram p17: hidden frame]
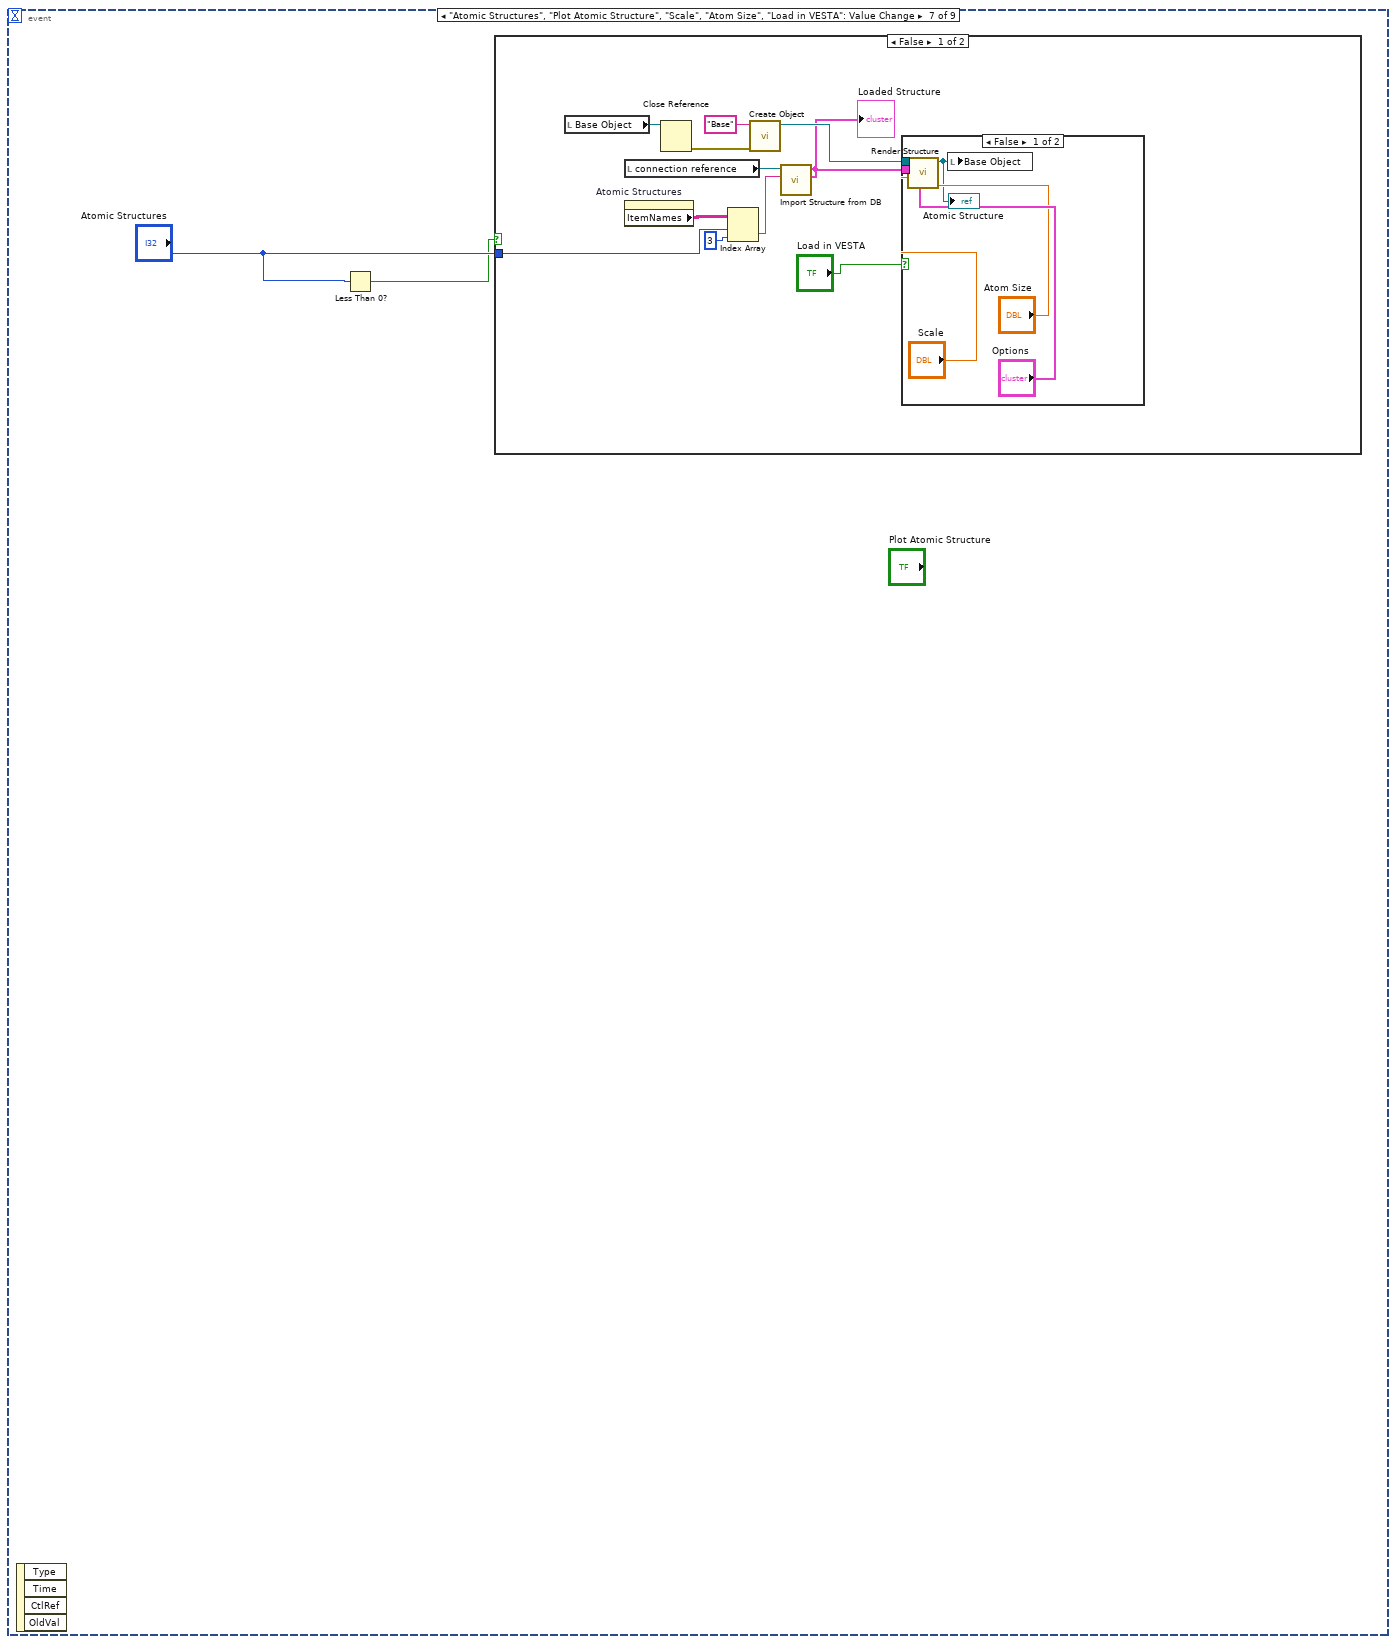
[diagram p18: hidden frame]
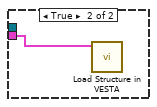
[diagram p19: hidden frame]
diagram:
  n1 = call-poly <vilib>:"DB Tools Open Connection.vi"("connection information"="UDL") -> ("error out"=w5:errorcluster, "connection reference"=w14:T5)  [unwired: 7 in]
  n2 = call-poly <vilib>:"DB Tools Execute Query.vi"("error in (no error)"=w5, "SQL query"="SELECT DISTINCT [0D_Point_Defects].Defect_Free_Structure_ID, [0D_Point_Defects].Defect_Free_Structure_Name, [0D_Point_Defects].[Defect_Free_Energy_(eV)]\nFROM [0D_Point_Defects];\n", "connection reference"=w14) -> ("error out"=w16:errorcluster, "recordset reference"=w13:T8)  [unwired: 5 in]
  n3 = call "Column Headers from SQL Query Recordset.vi"("error in (no error)"=w16, "recordset reference"=w13) -> ("error out"=w15:errorcluster, "columns"=w6:string[], "Recordset reference Out"=w12:T8)  [unwired: 6 in, 1 out]
  n4 = call-poly <vilib>:"DB Tools Fetch Recordset Data.vi"("error in (no error)"=w15, "recordset reference"=w12) -> ("error out"=w17:errorcluster, "recordset data"=w9:variant[][], "recordset reference out"=w11:T8)  [unwired: 3 in]
  n5 = for {
    tunnel: w9 -> [w20] mode=indexing
    tunnel: [w19] -> w8 mode=indexing
    n6 = for {
      tunnel: w20 -> [w23] mode=indexing
      tunnel: [w21] -> w19 mode=indexing
      n7 = xnode "Database Variant To Data"("database variant"=w23, "type"="") -> ("data"=w21:string)  [unwired: 1 in, 1 out]
    }
  }
  n8 = call-poly <vilib>:"DB Tools Free Object.vi"("error in (no error)"=w17, "recordset reference"=w11) -> ("connection reference"=→"connection reference":T5)  [unwired: 8 in, 1 out]
  n9 = call <vilib>:"Create Object.vi"("Name"="Base") -> ("error out"=w1:errorcluster, "Scene:New Object"=→"Base Object":refnum<vi>)  [unwired: 1 in, 8 out]
  n10 = property on="Pure Structures with defects" class="MCListbox (strict)"(error in=w1, "ColHdrString"=w6, "ItemNames"=w8) -> (error out=w4:errorcluster)  [unwired: 1 in, 1 out]
  n11 = while {
    tunnel: w4 -> [_]
    stop <- FALSE stop-if-true
    n12 = event shown="[1] \"Pure Structures with defects\", \"Chemical Potential\", \"Chemical Potential 2\", \"Thermodynamic Fermi Level\": Value Change" {
      selector: _ -> [_ _ _ _ _ _ _ _ _]
      dyn-events: _ -> [_ _ _ _ _ _ _ _ _]
      timeout: 60000 -> [_ _ _ _ _ _ _ _ _]
      event Timeout {
        n13 = event-data() -> ()  [unwired: 1 in, 2 out]
        n14 = Wait (ms)(milliseconds to wait=u32 10) -> ()  [unwired: 1 out]
      }
      event "Pure Structures with defects", "Chemical Potential", "Chemical Potential 2", "Thermodynamic Fermi Level": Value Change {
        w68 = -1.0 ("Thermodynamic Fermi Level (eV)")
        w74 = T10 {"Name"="Thermodynamic Fermi Level", "Color"=0, "Style"=2, "Point Style"=13, "Name Visible"=TRUE, "Allow Drag"=TRUE, "Cursor Mode"=0, "Plot"=0, "Index"=0, "Position"={"X"=2.4701149425287356, "Y"=0.0}, "X Scale"=0, "Y Scale"=0, "Watch Plots"=[], "Watch All Plots"=FALSE, "Plot Area"=0, "Label Offset"={"X"=0.016091954022988464, "Y"=2.3061224489795915}} ("element")
        n15 = event-data() -> ()  [unwired: 1 in, 3 out]
        n16 = local read "connection reference"() -> (w79:T5)
        n17 = property on="Pure Structures with defects" class="MCListbox (strict)"() -> ("ItemNames"=w83:string[][])  [unwired: 2 in, 2 out]
        n18 = Index Array(array=w83, index (col) #1=0 ("disabled index (col)")) -> (element #1=w80:string[], element #2=w62:string[])  [unwired: 3 in]
        n19 = for {
          tunnel: "Pure Structures with defects" -> [w90] mode=indexing
          tunnel: w80 -> [w116]
          shift-right: [w114] -> _
          shift-left: w79 -> [w115]
          shift-right: [w105] -> w61
          shift-left: string[][] [] -> [w104]
          tunnel: "Calc Thermodynamic Fermi Level" -> [w103]
          shift-right: [w110] -> w67
          shift-left: w68 -> [w100]
          shift-right: [w111] -> w66
          shift-left: w68 -> [w99]
          tunnel: [w97] -> w65 mode=indexing
          shift-right: [w93] -> w63
          shift-left: cluster{i32, i32}[] [] -> [w92]
          tunnel: w62 -> [w91]
          i -> [w95]
          n20 = Index Array(array=w116, index=w90) -> (element=w98:string)
          n21 = Index Array(array=w91, index=w90) -> (element=w89:string)
          n22 = property on="Pure Structures with defects" class="MCListbox (strict)"() -> ("ItemNames"=w109:string[][])  [unwired: 2 in, 2 out]
          n23 = local read "Volumes"() -> (w86:dbl[])
          n24 = local read "Chemical Potential 2"() -> (w112:dbl)
          n25 = local read "Chemical Potential"() -> (w113:dbl)
          n26 = Equal?(x="Thermodynamic Fermi Level", y=w90) -> (x = y?=w102:bool)
          n27 = call "DB Get Defects from pure ID.vi"("Ignore Location"="Ignore Location", "Defect Free Structure ID"=w98, "connection reference in"=w115) -> ("Defects Array"=w96:T11, "connection reference out"=w114:T5)  [unwired: 5 in, 2 out]
          n28 = Index Array(array=w109, index (row)=w90, index (col)=1 ("disabled index (col)")) -> (element=w107:string)
          n29 = Index Array(array=w86, index="Thermodynamic Fermi Level") -> (element=w85:dbl)
          n30 = for {
            tunnel: [w130] -> w106 mode=indexing
            tunnel: w107 -> [w129]
            tunnel: w96 -> [w128] mode=indexing
            tunnel: w95 -> [w126]
            tunnel: [w125] -> w94 mode=indexing
            i -> [w127]
            n31 = Unbundle By Name(w128) -> ("Defect Details"=w133:T12, "Charges and Energies"=w135:T13)
            n32 = Unbundle By Name(w133) -> ("Defect Name"=w132:string)
            n33 = for {
              tunnel: w135 -> [w141] mode=indexing
              shift-right: [w140] -> w131
              shift-left: "" -> [w139]
              n34 = Unbundle By Name(w141) -> ("Net Charge"=w138:i32)
              n35 = Number To Decimal String(number=w138) -> (decimal integer string=w137:string)  [unwired: 1 in]
              n36 = Concatenate Strings(w139, w137, ", " ("string")) -> (w140:string)
            }
            n37 = Build Array(w129, w132, w131) -> (w130:string[])
            n38 = Bundle(w126, w127) -> (w125:cluster{i32, i32})  [unwired: 1 in]
          }
          n39 = And(x=w103, y=w102) -> (x .and. y?=w101:bool)
          n40 = case shown="True" w101 {
            tunnel: w113 -> [_ w124]
            tunnel: w112 -> [_ w123]
            tunnel: [w117 w122] -> w111
            tunnel: [w118 w121] -> w110
            tunnel: w96 -> [_ w120]
            tunnel: w100 -> [w118 _]
            tunnel: w99 -> [w117 _]
            tunnel: w85 -> [_ w119]
            frame False {
            }
            frame True {
              n41 = call "Self-consistent charge neutrality.vi"("Volume (A³)"=w119, "Chemical Potential (0=Cd, 1=Te)"=w123, "Defects"=w120) -> ("Thermodynamic Fermi Level (eV) - VBM"=w121:dbl)  [unwired: 8 in]
              n42 = call "Self-consistent charge neutrality.vi"("Volume (A³)"=w119, "Chemical Potential (0=Cd, 1=Te)"=w124, "Defects"=w120) -> ("Thermodynamic Fermi Level (eV) - VBM"=w122:dbl)  [unwired: 8 in]
            }
          }
          n43 = Bundle(w89, "Defects Array"=w96) -> (w97:T14)  [unwired: 1 in]
          n44 = Build Array (concatenate)(w104, w106) -> (w105:string[][])
          n45 = Build Array (concatenate)(w92, w94) -> (w93:cluster{i32, i32}[])
        }
        "Thermodynamic Fermi Level (eV)" <- w66
        "All Hosts and Defects" <- w65
        "Indicies" <- w63
        n46 = disable-structure shown="Enabled" {
          disable-tunnel: [_ w84] -> w73
          frame Disabled {
          }
          frame Enabled {
            n47 = local read "Related Defects"() -> (w84:i32[])
          }
        }
        n48 = Index Array(array=w61, index (col)=1 ("disabled index (col)")) -> (element=w60:string[])  [unwired: 1 in]
        n49 = property on="Related Defects" class="MCListbox (strict)"("ColHdrString"=string[] ["Defect Free Structure", "Defect Name", "Net Charges"] ("Column Header Strings[]"), "ItemNames"=w61) -> (error out=w70:errorcluster)  [unwired: 2 in, 1 out]
        n50 = Bundle By Name(cluster=w74, "Position.X"=w67) -> (w75:T10)
        n51 = Bundle By Name(cluster=w74, "Position.X"=w66) -> (w77:T10)
        n52 = property on="Related Defects" class="MCListbox (strict)"(error in=w70, "Val(Sgnl)"=w73) -> ()  [unwired: 1 in, 2 out]
        n53 = Build Array(w75) -> (w76:T15)
        n54 = Build Array(w77) -> (w78:T15)
        n55 = property on="Defect" class="CmbBox"("Strings[]"=w60) -> ()  [unwired: 2 in, 2 out]
        n56 = property on="Te Rich Limit" class="XYGraph (strict)"("CrsrList"=w76) -> ()  [unwired: 2 in, 2 out]
        n57 = property on="Cd Rich Limit" class="XYGraph (strict)"("CrsrList"=w78) -> ()  [unwired: 2 in, 2 out]
      }
      event "Related Defects", "Show Charge Transitions", "Markov-Payne Correction": Value Change {
        w158 = T16 []
        n58 = event-data() -> ()  [unwired: 1 in, 4 out]
        n59 = local read "All Hosts and Defects"() -> (w148:T2)
        n60 = for {
          N -> [w197]
          tunnel: w148 -> [w183]
          tunnel: [w203] -> w153 mode=indexing
          tunnel: [w201] -> w155 mode=indexing
          tunnel: [w176] -> w145 mode=indexing
          tunnel: [w197] -> w162
          tunnel: "Related Defects" -> [w185] mode=indexing
          shift-right: [w191] -> w157
          shift-left: w158 -> [w195]
          tunnel: T9 {"Name"="0 / +1", "Color"=0, "Style"=4, "Point Style"=1, "Name Visible"=TRUE, "Allow Drag"=TRUE, "Annotation Mode"=0, "Plot"=-1, "Index"=0, "Position"={"X"=2.0, "Y"=1.0}, "X Scale"=0, "Y Scale"=0, "Show Arrow"=FALSE, "Lock Name"=FALSE, "Plot Area"=0, "Label Offset"={"X"=0.0, "Y"=0.05}} ("element 2") -> [w194]
          shift-right: [w190] -> w156
          shift-left: w158 -> [w192]
          tunnel: [w187] -> w150 mode=indexing
          shift-right: [w174] -> w146
          shift-left: string[][] [] -> [w173]
          n61 = local read "Indicies"() -> (w186:cluster{i32, i32}[])
          n62 = Index Array(array=w186, index=w185) -> (element=w184:cluster{i32, i32})
          n63 = local read "VBM"() -> (w169:dbl)
          n64 = call "Start and End to Array 2.vi"("Sweep Style"=enum16{"Linear Step", "Linear Pts", "Log Pts"}."Linear Pts", "Step or # Pts"=100.0, "End"=3.4, "Start"=w169) -> ("Array"=w193:dbl[])  [unwired: 7 in]
          n65 = Unbundle(w184) -> (w172:i32, w180:i32)
          n66 = Index Array(array="Volumes", index=w172) -> (element=w170:dbl)
          n67 = Index Array(array=w183, index=w172) -> (element=w182:T17)
          n68 = Build Array (concatenate)(w193) -> (w189:dbl[])
          n69 = Unbundle(w182) -> ("Defect Free Name"=w177:string, "Defects Array"=w181:T11)
          n70 = Index Array(array=w181, index=w180) -> (element=w179:T18)
          n71 = Unbundle By Name(w179) -> ("Defect Details.Defect Name"=w176:string, "Charges and Energies"=w178:T13)
          n72 = case shown="True" "Show Charge Transitions" {
            tunnel: w179 -> [_ w226]
            tunnel: w195 -> [_ w224]
            tunnel: w194 -> [_ w225]
            tunnel: w192 -> [_ w221]
            tunnel: [_ w222] -> w191
            tunnel: [_ w219] -> w190
            tunnel: w176 -> [_ w217]
            tunnel: [_ w216] -> w187
            tunnel: w170 -> [_ w215]
            frame False {
            }
            frame True {
              n73 = local read "VBM"() -> (w213:dbl)
              n74 = local read "Markov-Payne Correction"() -> (w214:bool)
              n75 = call "Find Charge Transitions.vi"("Dielectric Constant"=11.0, "Volume (A³)"=w215, "Markov-Payne Corrections"=w214, "VBM"=w213, "Defect Data"=w226) -> ("Transitions"=w218:T3)  [unwired: 6 in]
              "Transitions" <- w218
              n76 = for {
                tunnel: w218 -> [w241] mode=indexing
                tunnel: w225 -> [w239]
                tunnel: [w235] -> w223 mode=indexing
                tunnel: [w234] -> w220 mode=indexing
                n77 = local read "Chemical Potential 2"() -> (w228:dbl)
                n78 = local read "Chemical Potential"() -> (w231:dbl)
                n79 = Unbundle(w241) -> ("Transition"=w238:string, "Fermi Energy (eV)"=w237:dbl, "Formation Energy, Cd Rich (eV)"=w233:dbl, "Formation Energy, Te Rich (eV)"=w232:dbl)
                n80 = Build Array(w233, w232) -> (w229:dbl[])
                n81 = Interpolate 1D Array(1:w231, 2:w229) -> (0:w230:dbl)
                n82 = Interpolate 1D Array(1:w228, 2:w229) -> (0:w227:dbl)
                n83 = Bundle("Fermi Energy (eV)"=w237, w230) -> (w240:cluster{"Fermi Energy (eV)":dbl, dbl})  [unwired: 1 in]
                n84 = Bundle("Fermi Energy (eV)"=w237, w227) -> (w236:cluster{"Fermi Energy (eV)":dbl, dbl})  [unwired: 1 in]
                n85 = Bundle By Name(cluster=w239, "Name"=w238, "Position"=w240) -> (w235:T9)
                n86 = Bundle By Name(cluster=w239, "Name"=w238, "Position"=w236) -> (w234:T9)
              }
              n87 = Bundle("Defect Name"=w217, "Transitions"=w218) -> (w216:T19)  [unwired: 1 in]
              n88 = Build Array (concatenate)(w224, w223) -> (w222:T16)
              n89 = Build Array (concatenate)(w221, w220) -> (w219:T16)
            }
          }
          n90 = for {
            tunnel: w189 -> [w248] mode=indexing
            tunnel: [w247] -> w204 mode=indexing
            tunnel: [w246] -> w202 mode=indexing
            tunnel: w179 -> [w245]
            tunnel: w170 -> [w243]
            w242 = 11.0 ("Dielectric Constant")
            n91 = call "Calc Formation Energy from Defect Cluster.vi"("Dielectric Constant"=w242, "Volume (A³)"=w243, "Markov-Payne Correction"="Markov-Payne Correction", "Chemical Potential"="Chemical Potential 2", "Fermi Level (eV)"=w248, "Defect Data"=w245) -> ("Formation Energy (eV)"=w246:dbl)  [unwired: 4 in, 1 out]
            n92 = call "Calc Formation Energy from Defect Cluster.vi"("Dielectric Constant"=w242, "Volume (A³)"=w243, "Markov-Payne Correction"="Markov-Payne Correction", "Chemical Potential"="Chemical Potential", "Fermi Level (eV)"=w248, "Defect Data"=w245) -> ("Formation Energy (eV)"=w247:dbl)  [unwired: 4 in, 1 out]
          }
          n93 = for {
            tunnel: w178 -> [w211] mode=indexing
            tunnel: w177 -> [w208]
            tunnel: w176 -> [w207]
            tunnel: [w206] -> w175 mode=indexing
            n94 = Unbundle By Name(w211) -> ("Net Charge"=w210:i32, "Structure ID"=w205:string)
            n95 = Number To Decimal String(number=w210) -> (decimal integer string=w209:string)  [unwired: 1 in]
            n96 = Build Array(w208, w207, w209, w205) -> (w206:string[])
          }
          n97 = Build Array (concatenate)(w173, w175) -> (w174:string[][])
          n98 = Subtract(x=w189, y=w169) -> (x-y=w188:dbl[])
          n99 = Bundle(w188, w202) -> (w201:cluster{dbl[], dbl[]})  [unwired: 1 in]
          n100 = Bundle(w188, w204) -> (w203:cluster{dbl[], dbl[]})  [unwired: 1 in]
        }
        "Cd Rich Limit" <- w153
        "Te Rich Limit" <- w155
        n101 = local read "Plots Tab"() -> (w154:T6)
        n102 = case shown="\"Binding Energy\"" w154 {
          frame "Formation Energies vs Fermi", Default {
          }
          frame "Binding Energy" {
            n103 = property on="Plot Binding Energy" class="Bool (strict)"("Val(Sgnl)"=TRUE ("Value (Signaling)")) -> ()  [unwired: 2 in, 2 out]
          }
          frame "Charge Transition Levels" {
          }
          frame "Atomic Structure" {
          }
        }
        n104 = property on="Atomic Structures" class="MCListbox (strict)"("ItemNames"=w146) -> ()  [unwired: 2 in, 2 out]
        n105 = property on="Te Rich Limit" class="XYGraph (strict)"("AnntList"=w156) -> ()  [unwired: 2 in, 2 out]
        n106 = property on="Cd Rich Limit" class="XYGraph (strict)"("AnntList"=w157) -> ()  [unwired: 2 in, 2 out]
        n107 = control-ref of="Defect Energy Levels"() -> (w151:refnum<vi>)
        n108 = disable-structure shown="Enabled" {
          disable-tunnel: w150 -> [w164 w167]
          disable-tunnel: [w163 w167] -> w149
          frame Disabled {
            n109 = Decimate 1D Array(w164) -> (w166:T20, w165:T20)
            n110 = Build Array (concatenate)(w166, w165) -> (w163:T20)
          }
          frame Enabled {
          }
        }
        n111 = call "Make Defect Energy Transition Plot.vi"("Buckets"="Buckets", "All Defects and Transitions"=w149, "XY Graph Reference"=w151) -> ()  [unwired: 9 in]
        n112 = call "Num of Colors to Color Array.vi"("# of Colors"=w162, "Color Array Type"="Color Array Type") -> ("Colors Array"=w143:u32[])  [unwired: 3 in]
        n113 = control-ref of="Te Rich Limit"() -> (w152:refnum<vi>)
        n114 = control-ref of="Cd Rich Limit"() -> (w161:refnum<vi>)
        n115 = call "Format XY Plot.vi"("Colors Array"=w143, "Plot Names"=w145, "XY Graph Reference"=w152) -> ()  [unwired: 9 in]
        n116 = call "Format XY Plot.vi"("Colors Array"=w143, "Plot Names"=w145, "XY Graph Reference"=w161) -> ()  [unwired: 9 in]
      }
      event "Save as a table": Value Change {
        n117 = event-data() -> ()  [unwired: 1 in, 4 out]
        n118 = call "Fermi Level?"() -> ("Fermi Level"=w251:dbl, "OK"=w252:bool)  [unwired: 17 in, 1 out]
        n119 = case shown="True" w252 {
          tunnel: w251 -> [_ w260]
          frame False {
          }
          frame True {
            n120 = Less Or Equal To 0?(x=w260) -> (x <= 0?=w261:bool)
            n121 = local read "All Hosts and Defects"() -> (w253:T2)
            n122 = case shown="False" w261 {
              tunnel: [w278 w279] -> w254
              tunnel: w260 -> [w278 _]
              frame False {
              }
              frame True {
                n123 = local read "Thermodynamic Fermi Level (eV)"() -> (w279:dbl)
              }
            }
            n124 = local read "Related Defects"() -> (w277:i32[])
            n125 = Add(x="VBM", y=w254) -> (x+y=w266:dbl)
            n126 = for {
              tunnel: w277 -> [w282] mode=indexing
              tunnel: [w294] -> w276 mode=indexing
              tunnel: [w293] -> w275 mode=indexing
              tunnel: w266 -> [w292]
              tunnel: [w291] -> w259 mode=indexing
              tunnel: [w289] -> w257 mode=indexing
              tunnel: w253 -> [w283]
              n127 = local read "Chemical Potential"() -> (w295:dbl)
              n128 = local read "Indicies"() -> (w288:cluster{i32, i32}[])
              n129 = Index Array(array=w288, index=w282) -> (element=w287:cluster{i32, i32})
              n130 = Unbundle(w287) -> (w286:i32, w284:i32)
              n131 = Index Array(array=w283, index=w286) -> (element=w285:T17)
              n132 = Unbundle(w285) -> ("Defects Array"=w281:T11)  [unwired: 1 out]
              n133 = Index Array(array=w281, index=w284) -> (element=w280:T18)
              n134 = call "Calc Formation Energy from Defect Cluster.vi"("Chemical Potential"=w295, "Fermi Level (eV)"=w292, "Defect Data"=w280) -> ("Net Charge"=w291:i32, "Formation Energy (eV)"=w294:dbl)  [unwired: 7 in]
              n135 = Unbundle By Name(w280) -> ("Defect Details.Defect Name"=w293:string, "Defect Details.Reference Pure Structure Energy"=w290:dbl)
              n136 = Number To Fractional String(number=w290) -> (F-format string=w289:string)  [unwired: 3 in]
            }
            n137 = Number To Fractional String(number="VBM") -> (F-format string=w255:string)  [unwired: 3 in]
            n138 = local read "Chemical Potential"() -> (w271:dbl)
            n139 = Number To Fractional String(number=w271) -> (F-format string=w270:string)  [unwired: 3 in]
            n140 = Number To Fractional String(number=w254) -> (F-format string=w272:string)  [unwired: 3 in]
            n141 = Number To Fractional String(number=w276) -> (F-format string=w274:string[])  [unwired: 3 in]
            n142 = Build Array(w270, w272, w255) -> (w268:string[])
            n143 = Number To Decimal String(number=w259) -> (decimal integer string=w258:string[])  [unwired: 1 in]
            n144 = Build Array(w275, w257, w274, w258) -> (w273:string[][])
            n145 = Build Array(string[] ["Chemical Potential (% Te Rich)", "Fermi Energy (eV)", "VBM"], w268) -> (w267:string[][])
            n146 = Transpose 2D Array(2D array=w273) -> (transposed array=w263:string[][])
            n147 = Build Array (concatenate)(w267, string[] [" "] ("element"), string[] ["Defect Name", "Defect Free Energy", "Formation Energy (eV)", "Net Charge"], w263) -> (w265:string[][])
            n148 = call-poly <vilib>:"Write To Spreadsheet File.vi"("2D data"=w265) -> ()  [unwired: 7 in, 1 out]
          }
        }
      }
      event "Set as seperate defects": Value Change {
        n149 = event-data() -> ()  [unwired: 1 in, 4 out]
        n150 = local read "Related Defects"() -> (→"Defects to Bind":i32[])
        n151 = property on="Related Defects" class="MCListbox (strict)"() -> ("Value"=w299:i32[], "ItemNames"=w298:string[][])  [unwired: 2 in, 2 out]
        n152 = for {
          tunnel: w299 -> [w303] mode=indexing
          tunnel: w298 -> [w302]
          tunnel: [w300] -> w297 mode=indexing
          n153 = Index Array(array=w302, index (row)=w303, index (col)=1 ("disabled index (col)")) -> (element=w300:string)
        }
        n154 = property on="Seperate Defects" class="LstBox (strict)"("Item Names"=w297) -> ()  [unwired: 2 in, 2 out]
      }
      event "Plot Binding Energy": Value Change {
        w324 = 1.79581 ("Start")
        n155 = event-data() -> ()  [unwired: 1 in, 4 out]
        n156 = local read "All Hosts and Defects"() -> (w304:T2)
        n157 = local read "Defects to Bind"() -> (w338:i32[])
        n158 = call "Start and End to Array 2.vi"("Sweep Style"=enum16{"Linear Step", "Linear Pts", "Log Pts"}."Linear Pts", "Step or # Pts"=30.0, "End"=3.4, "Start"=w324) -> ("Array"=w322:dbl[])  [unwired: 7 in]
        n159 = for {
          N -> [w369]
          tunnel: [w369] -> _
          tunnel: w338 -> [w367]
          tunnel: w322 -> [w368] mode=indexing
          tunnel: [w365] -> w332 mode=indexing
          tunnel: "Binding Energy Chem Pot" -> [w364]
          tunnel: w304 -> [w363]
          n160 = for {
            tunnel: w368 -> [w384]
            tunnel: [w382] -> w366 mode=indexing
            tunnel: w367 -> [w375] mode=indexing
            tunnel: w364 -> [w383]
            tunnel: w363 -> [w376]
            n161 = local read "Markov-Payne Correction"() -> (w373:bool)
            n162 = local read "Indicies"() -> (w377:cluster{i32, i32}[])
            n163 = local read "Volumes"() -> (w372:dbl[])
            n164 = Index Array(array=w377, index=w375) -> (element=w378:cluster{i32, i32})
            n165 = Unbundle(w378) -> (w371:i32, w380:i32)
            n166 = Index Array(array=w372, index=w371) -> (element=w370:dbl)
            n167 = Index Array(array=w376, index=w371) -> (element=w379:T17)
            n168 = Unbundle(w379) -> ("Defects Array"=w381:T11)  [unwired: 1 out]
            n169 = Index Array(array=w381, index=w380) -> (element=w374:T18)
            n170 = call "Calc Formation Energy from Defect Cluster.vi"("Volume (A³)"=w370, "Markov-Payne Correction"=w373, "Chemical Potential"=w383, "Fermi Level (eV)"=w384, "Defect Data"=w374) -> ("Formation Energy (eV)"=w382:dbl)  [unwired: 5 in, 1 out]
          }
          n171 = Add Array Elements(numeric array=w366) -> (sum=w365:dbl)
        }
        n172 = local read "Related Defects"() -> (w334:i32[])
        n173 = Subtract(x=w322, y=w324) -> (x-y=w323:dbl[])
        n174 = Bundle(w323, w332) -> (w333:cluster{dbl[], dbl[]})  [unwired: 1 in]
        n175 = for {
          tunnel: w334 -> [w340] mode=indexing
          tunnel: [w358] -> w329 mode=indexing
          tunnel: w323 -> [w357]
          tunnel: [w356] -> w328 mode=indexing
          tunnel: w332 -> [w354]
          tunnel: "Binding Energy Chem Pot" -> [w352]
          tunnel: [w350] -> w326 mode=indexing
          tunnel: [w349] -> w316 mode=indexing
          tunnel: w322 -> [w348]
          tunnel: w304 -> [w341]
          n176 = local read "Indicies"() -> (w342:cluster{i32, i32}[])
          n177 = Index Array(array=w342, index=w340) -> (element=w343:cluster{i32, i32})
          n178 = Unbundle(w343) -> (w344:i32, w346:i32)
          n179 = Index Array(array=w341, index=w344) -> (element=w345:T17)
          n180 = Unbundle(w345) -> ("Defects Array"=w347:T11)  [unwired: 1 out]
          n181 = Index Array(array=w347, index=w346) -> (element=w339:T18)
          n182 = Unbundle By Name(w339) -> ("Defect Details.Defect Name"=w349:string)
          n183 = for {
            tunnel: w348 -> [w362] mode=indexing
            tunnel: [w361] -> w355 mode=indexing
            tunnel: w352 -> [w360]
            tunnel: w339 -> [w359]
            n184 = call "Calc Formation Energy from Defect Cluster.vi"("Chemical Potential"=w360, "Fermi Level (eV)"=w362, "Defect Data"=w359) -> ("Formation Energy (eV)"=w361:dbl)  [unwired: 7 in, 1 out]
          }
          n185 = Subtract(x=w355, y=w354) -> (x-y=w353:dbl[])
          n186 = Concatenate Strings("Binding of " ("string"), w349) -> (w350:string)
          n187 = Bundle(w357, w353) -> (w356:cluster{dbl[], dbl[]})  [unwired: 1 in]
          n188 = Bundle(w357, w355) -> (w358:cluster{dbl[], dbl[]})  [unwired: 1 in]
        }
        n189 = local read "Color Array Type"() -> (w319:T4)
        n190 = Interleave 1D Arrays(w329, w328) -> (w327:cluster{dbl[], dbl[]}[])
        n191 = Interleave 1D Arrays(w316, w326) -> (w320:string[])
        n192 = Array Size(array=w316) -> (size(s)=w310:i32)
        n193 = Build Array (concatenate)(w333, w327) -> (→"Binding Energy":cluster{dbl[], dbl[]}[])
        n194 = call "Num of Colors to Color Array.vi"("# of Colors"=w310, "Color Array Type"=w319) -> ("Colors Array"=w315:u32[])  [unwired: 3 in]
        n195 = Initialize Array(0, w310) -> (w308:i32[])
        n196 = Initialize Array(1, w310) -> (w307:i32[])
        n197 = Build Array (concatenate)("Seperate" ("String"), w320) -> (w321:string[])
        n198 = Interleave 1D Arrays(w315, w315) -> (w314:u32[])
        n199 = Interleave 1D Arrays(w308, w307) -> (w306:i32[])
        n200 = control-ref of="Binding Energy"() -> (w313:refnum<vi>)
        n201 = Build Array (concatenate)(0, w306) -> (w305:i32[])
        n202 = Build Array (concatenate)(u32 0 ("Color Box"), w314) -> (w317:u32[])
        n203 = call "Format XY Plot.vi"("Active Y Scale (Left or Right)"=w305, "Line Styles"=w305, "Colors Array"=w317, "Plot Names"=w321, "XY Graph Reference"=w313) -> ()  [unwired: 7 in]
      }
      event "Atomic Structures", "Plot Atomic Structure", "Scale", "Atom Size", "Load in VESTA": Value Change {
        n204 = event-data() -> ()  [unwired: 1 in, 4 out]
        n205 = Less Than 0?(x="Atomic Structures") -> (x < 0?=w385:bool)
        n206 = case shown="False" w385 {
          tunnel: "Atomic Structures" -> [w389 _]
          frame False {
            n207 = local read "Base Object"() -> (w395:refnum<vi>)
            n208 = local read "connection reference"() -> (w390:T5)
            n209 = property on="Atomic Structures" class="MCListbox (strict)"() -> ("ItemNames"=w393:string[][])  [unwired: 2 in, 2 out]
            n210 = Close Reference(reference=w395) -> (error out=w394:errorcluster)  [unwired: 1 in]
            n211 = Index Array(array=w393, index (row)=w389, index (col)=3 ("disabled index (col)")) -> (element=w391:string)
            n212 = call <vilib>:"Create Object.vi"("error in (no error)"=w394, "Name"="Base") -> ("Scene:New Object"=w396:refnum<vi>)  [unwired: 9 out]
            n213 = call "Import Structure from DB.vi"("Structure ID"=w391, "connection reference"=w390) -> ("Loaded Structure"=w388:T1)  [unwired: 7 in, 2 out]
            "Loaded Structure" <- w388
            n214 = case shown="False" "Load in VESTA" {
              tunnel: w396 -> [w401 _]
              tunnel: w388 -> [w398 w404]
              frame False {
                n215 = call "Render Structure.vi"("Options"="Options", "Atom Size"="Atom Size", "Scale"="Scale", "Atomic Structure"=w398, "Base Object"=w401) -> ("Object with atoms"=w400:refnum<vi>)  [unwired: 6 in]
                "Atomic Structure" <- w400
                n216 = local write "Base Object"(w400) -> ()
              }
              frame True {
                n217 = call "Load Structure in VESTA.vi"("Atomic Structure"=w404) -> ()  [unwired: 11 in]
              }
            }
          }
          frame True {
          }
        }
      }
      event "Setup Camera": Value Change {
        n218 = event-data() -> ()  [unwired: 1 in, 4 out]
        n219 = local read "Loaded Structure"() -> (w420:T1)
        n220 = Unbundle By Name(w420) -> ("Lattice vector a"=w410:dbl[], "Lattice vector b"=w409:dbl[], "Lattice vector c"=w419:dbl[])
        n221 = control-ref of="Atomic Structure"() -> (w405:refnum<vi>)
        n222 = Negate(x=w410) -> (-x=w408:dbl[])
        n223 = Compound Arithmetic op=ADD(w410, w409, w419) -> (w417:dbl[])
        n224 = local read "Scale"() -> (w416:dbl)
        n225 = Divide(x=w417, y=2.0) -> (x/y=w415:dbl[])
        n226 = Multiply(x=w415, y=w416) -> (x*y=w414:dbl[])
        n227 = Multiply(x=w408, y=2.0 ("Numeric")) -> (x*y=w406:dbl[])
        n228 = Array To Cluster(array=w406) -> (cluster=w411:cluster{"[0]":dbl, "[1]":dbl, "[2]":dbl})
        n229 = Array To Cluster(array=w414) -> (cluster=w413:cluster{"[0]":dbl, "[1]":dbl, "[2]":dbl})
        n230 = Array To Cluster(array=w409) -> (cluster=w412:T21)
        n231 = invoke on="Invoke Node" class="SceneGraphDisp (strict)" method="Setup Camera"(reference=w405, "Camera Position"=w411, "Target"=w413, "Up Direction"=w412) -> ()  [unwired: 2 in, 6 out]
      }
      event "Make Awesome Looking": Value Change {
        n232 = event-data() -> ()  [unwired: 1 in, 4 out]
        n233 = control-ref of="Cd Rich Limit"() -> (w426:refnum<vi>)
        n234 = local read "Defect Energy Levels"() -> (w427:cluster{dbl[], dbl[]}[])
        n235 = local read "Cd Rich Limit"() -> (w423:cluster{"appended array":dbl[], dbl[]}[])
        n236 = local read "Te Rich Limit"() -> (w428:cluster{dbl[], dbl[]}[])
        n237 = property on="Defect Energy Levels" class="XYGraph (strict)"() -> ("AnntList"=w421:T22)  [unwired: 2 in, 2 out]
        n238 = Array Size(array=w423) -> (size(s)=w422:i32)
        n239 = for {
          N: w422 -> [_]
          tunnel: w426 -> [w432]
          tunnel: [w430] -> w425 mode=indexing
          tunnel: [w429] -> w424 mode=indexing
          i -> [w431]
          n240 = property on="Property Node" class="XYGraph (strict)"(reference=w432, "Active Plot"=w431) -> ("Plot.Plot Color"=w430:u32, "Plot.Plot Name"=w429:string)  [unwired: 1 in, 2 out]
        }
        n241 = call "Awesome Looking Plots for Defect Buddy.vi"("Colors Array"=w425, "Plot Names"=w424, "Annotation List for Charge States"=w421, "Defect Energy Levels"=w427, "Te Rich Limit"=w428, "Cd Rich Limit"=w423) -> ()  [unwired: 6 in]
      }
    }
  }
  n242 = disable-structure shown="Disabled" {
    frame Disabled {
    }
    frame Enabled {
    }
  }
  n243 = disable-structure shown="Disabled" {
    frame Disabled {
      n244 = for {
        N: 9 -> [_]
        i -> [w442]
        n245 = control-ref of="Te Rich Limit"() -> (w436:refnum<vi>)
        n246 = property on="Property Node" class="XYGraph (strict)"(reference=w436, "Active Plot"=w442) -> ("Plot.Point Style"=w441:u8, "Plot.Fill/Pt. Color"=w440:u32, "Plot.Plot Color"=w439:u32, "Plot.Plot Interpolation"=w438:u8, "Plot.Line Width"=w437:u8, "Plot.Line Style"=w434:u8)  [unwired: 1 in, 2 out]
        n247 = control-ref of="Cd Rich Limit"() -> (w435:refnum<vi>)
        n248 = property on="Property Node" class="XYGraph (strict)"(reference=w435, "Active Plot"=w442, "Plot.Point Style"=w441, "Plot.Fill/Pt. Color"=w440, "Plot.Plot Color"=w439, "Plot.Plot Interpolation"=w438, "Plot.Line Width"=w437, "Plot.Line Style"=w434) -> ()  [unwired: 1 in, 2 out]
      }
    }
    frame Enabled {
    }
  }
